vi "SDS Process Mngr.vi"(0 "State In":T5, 1 "Mngr Action":T12, 2 "FP":T11, 7 "Cartridges":T4, 9 "Manual Input":dbl format="%#_13g", 11 "error in (no error)":errorcluster, 12 "Config":T1={"Syringe size"=0, "Syringe address"=0, "# of ports"=0, "Init String"="Z0N1R", "Full Stroke (cnts)"=0, "Model"=enum."XC", "TW Position"=0.0, "Load Position"=0.0, "Bottom Position"=0.0, "Station ID"="", "Default Protocol"=path "", "Dry Time(s)"=0.0, "Python Version"="", "NFC SN Array"=["21121521200223", "21121521200186", "21121521200213", "52541737200062"], "Timing"={"Checking pres and leak"=0.0, "Priming input lines"=0.0, "Rinsing syringe"=0.0, "Filling well X w/ X"=0.0, "Drain well X"=0.0, "Clearing wells and lines"=0.0, "Draining wells"=0.0, "Rinsing all wells"=0.0, "Testing for leaks/clogs"=0.0, "Rinsing wells"=0.0}, "Pressure Specs"={"Pressure max"=0.0, "Pressure min"=0.0, "Decay delta"=0.0, "Pressure time"=0.0, "Conf. R"=0.0, "LeakRateMax"=0.0}}) -> (6 "State Out":T5, 15 "error out":errorcluster)   [LabVIEW 2020]
uses:
  Process Mngr.ctl
  Main Refs.ctl
  Wash Step.ctl
  Process State.ctl
  Results.ctl
  Vacuum Test.ctl
  Pressure Output.ctl
  Cartridge #.ctl
  Hardware/Tecan/Pump Config.ctl
  Timing Specs.ctl
  Vacuum Specs.ctl
  status update.ctl
  Cartridge Mngr.ctl
  Time elapsed.ctl
  Hardware/DAQ Mngr.ctl
  Lib/Time/Bottles.ctl
  Hardware/Mot Stage Mngr.ctl
  Update Single Cart.ctl
  Hardware/16CH Denkovi Mngr.ctl
  Hardware/Tricon Mngr.ctl
  Hardware/Tecan/Pump Control.ctl
  Pump Port.ctl
  Hardware/Tecan/Velocity Units.ctl
  Main Globals.vi
  Lib/Utilities.lvlib
panel:
  out "Reports":T6[](array[typedef])
  in  "Pressure Specs":T9
  out "Wash Array":T10[](array[typedef]) {"# of Rinses" max=10}
  # "Tecan Pump"
  # "Pressure"
  # "General"
  # "Timing"
  # "Protocol"
  # "Zaber"
  # "NFC Reader 1"
  # "NFC  Reader 2"
  # "NFC Reader 3"
  # "NFC Reader 4"
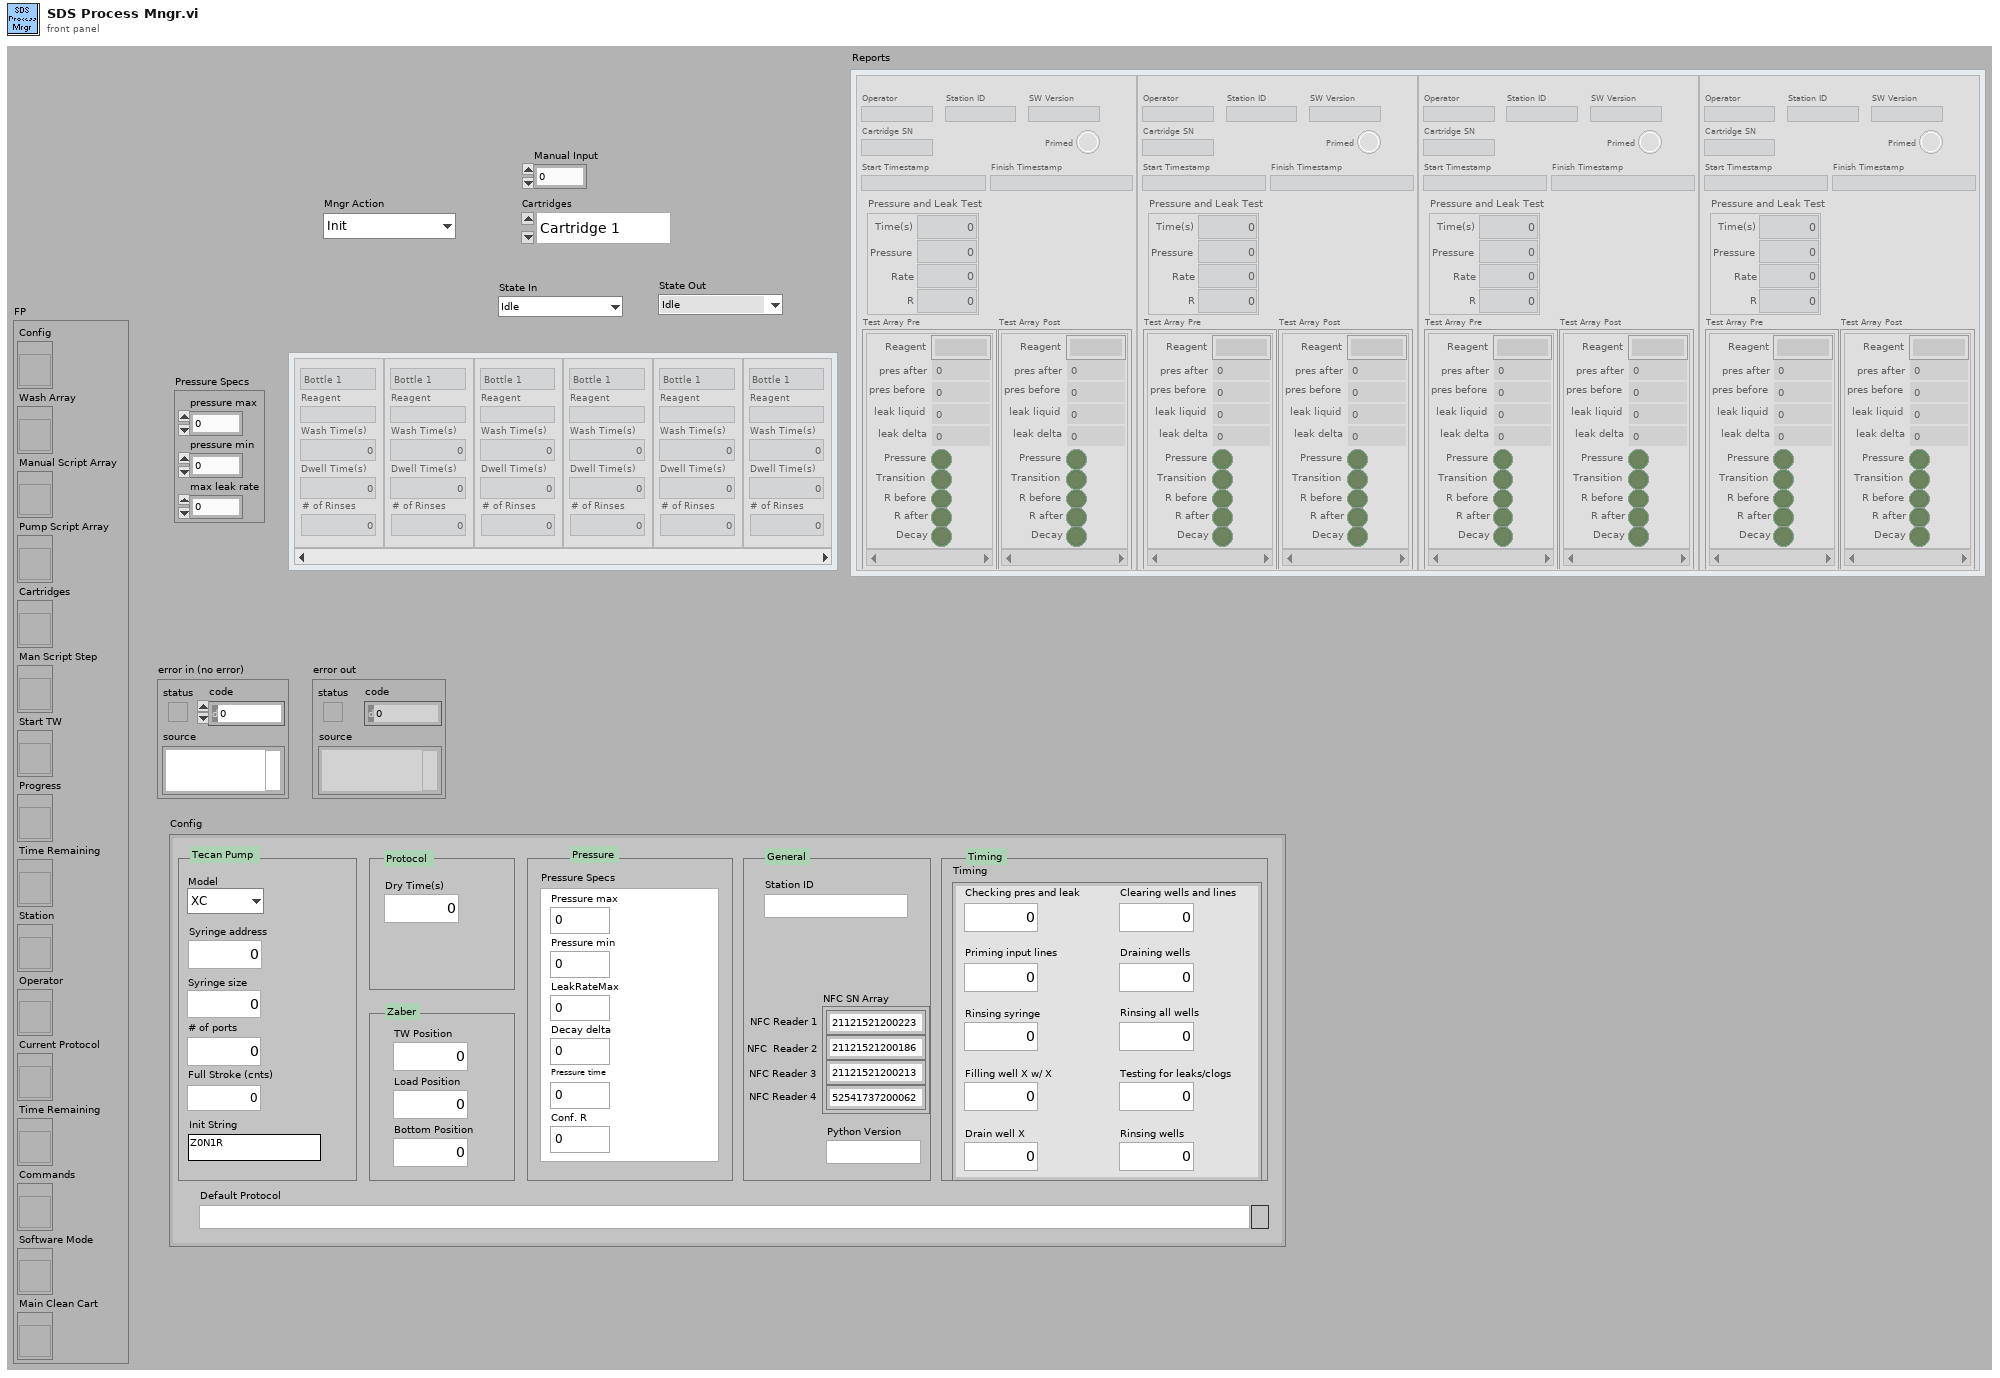
[diagram p1: front panel]
types:
  T1 = typedef "Pump Config.ctl" = cluster{"Syringe size":u32, "Syringe address":u32, "# of ports":u32, "Init String":string, "Full Stroke (cnts)":i32, "Model":enum16{"XC", "Centris"}, "TW Position":dbl, "Load Position":dbl, "Bottom Position":dbl, "Station ID":string, "Default Protocol":path, "Dry Time(s)":dbl, "Python Version":string, "NFC SN Array":string[], "Timing":T2, "Pressure Specs":T3}
  T2 = typedef "Timing Specs.ctl" = cluster{"Checking pres and leak":dbl, "Priming input lines":dbl, "Rinsing syringe":dbl, "Filling well X w/ X":dbl, "Drain well X":dbl, "Clearing wells and lines":dbl, "Draining wells":dbl, "Rinsing all wells":dbl, "Testing for leaks/clogs":dbl, "Rinsing wells":dbl}
  T3 = typedef "Vacuum Specs.ctl" = cluster{"Pressure max":dbl, "Pressure min":dbl, "Decay delta":dbl, "Pressure time":dbl, "Conf. R":dbl, "LeakRateMax":dbl}
  T4 = typedef "Cartridge #.ctl" = enum16{"Cartridge 1", "Cartridge 2", "Cartridge 3", "Cartridge 4"}
  T5 = typedef "Process State.ctl" = enum16{"Idle", "Init", "Check for SN", "Start TW", "SystemLeakTest", "Prime System", "Rinse Wells", "Fill Wells", "PrePresTest", "Apply Pressure", "PostPresTest", "Drain&Rinse", "Dry", "Report", "Finish", "Abort", "Error", "-rinse wells", "-check cartridge", "-clean cartridge", "-drain all", "-fill well"}
  T6 = typedef "Results.ctl" = cluster{"Operator":string, "Station ID":string, "SW Version":string, "Cartridge SN":string, "Primed":bool, "Start Timestamp":string, "Finish Timestamp":string, "Test Array Pre":T7[], "Test Array Post":T7[], "Pressure and Leak Test":T8}
  T7 = typedef "Vacuum Test.ctl" = cluster{"pres after":dbl, "pres before":dbl, "leak liquid":dbl, "leak delta":dbl, "Transition":bool, "Pressure":bool, "R before":bool, "R after":bool, "Reagent":string, "Decay":bool}
  T8 = typedef "Pressure Output.ctl" = cluster{"Time(s)":dbl, "Pressure":dbl, "Rate":dbl, "R":dbl}
  T9 = cluster{"pressure max":dbl, "pressure min":dbl, "max leak rate":dbl}
  T10 = typedef "Wash Step.ctl" = cluster{"Reagent":string, "Bottle":enum16{"Bottle 1", "Bottle 2", "Bottle 3", "Bottle 4"}, "Wash Time(s)":dbl, "Dwell Time(s)":dbl, "# of Rinses":i16}
  T11 = typedef "Main Refs.ctl" = cluster{"Config":refnum<vi>, "Wash Array":refnum<vi>, "Manual Script Array":refnum<vi>, "Pump Script Array":refnum<vi>, "Cartridges":refnum<vi>, "Man Script Step":refnum<vi>, "Start TW":refnum<vi>, "Progress":refnum<vi>, "Time Remaining":refnum<vi>, "Station":refnum<vi>, "Operator":refnum<vi>, "Current Protocol":refnum<vi>, "Time Remaining":refnum<vi>, "Commands":refnum<vi>, "Software Mode":refnum<vi>, "Main Clean Cart":refnum<vi>}
  T12 = typedef "Process Mngr.ctl" = enum16{"Init", "Run Step", "Update"}
  T13 = enum8{"Enabled", "Disabled", "Disabled and Grayed Out"}
  T14 = typedef "status update.ctl" = enum16{"Cartridge", "Main Status", "Reagent"}
  T15 = typedef "Cartridge Mngr.ctl" = enum16{"Init", "Update", "Detect", "Lock", "Read SN", "Unlock", "Error"}
  T16 = enum16{"Init Pressure", "Init Vacuum", "Save Pressure", "Save Vacuum", "Close"}
  T17 = typedef "DAQ Mngr.ctl" = enum16{"Init", "Read Pressure", "Read Vacuum", "Analyze Pres&Vac", "Analyze Vacuum", "Read Cartridges", "Lock Cartridge", "Unlock Cartridge", "Read PS", "Pinch Valve Engage", "Pinch Valve Disengage", "Close"}
  T18 = typedef "Time elapsed.ctl" = enum16{"Start", "Update", "Read"}
  T19 = typedef "Bottles.ctl" = enum16{"Bottle 1", "Bottle 2", "Bottle 3", "H2O", "Waste"}
  T20 = typedef "Mot Stage Mngr.ctl" = enum16{"Connect", "Init", "Status", "Send Cmd", "Current Pos", "Set Accel", "Set Max Vel", "Home", "Rel Move", "Abs Move", "Close"}
  T21 = typedef "Update Single Cart.ctl" = enum16{"Cart Status", "Cart Reagent"}
  T22 = typedef "16CH Denkovi Mngr.ctl" = enum16{"Search", "Init", "Set Peristaltic", "Set Pressure", "Set Vacuum", "Set PresVac", "Pres Vent&Close", "Vac Vent&Close", "Pres ON", "Vac ON", "Set All Relays", "Set One Relay", "Read Relays", "Close"}
  T23 = typedef "Pump Control.ctl" = cluster{"Syringe Pos":u32, "Rate":dbl, "Volume":dbl, "Valve":T24, "Action":enum32{"Withdraw", "Dispense", "Stop"}, "Move Type":enum32{"Abs", "Rel"}, "Init":bool, "Empty Syr.":bool, "Full Fill":bool, "Units":T25}
  T24 = typedef "Pump Port.ctl" = enum16{"Bottle 1", "Bottle 2", "Bottle 3", "Bottle 4", "Waste", "Well 1", "Well 2", "Well 3", "Well 4", "Bottle X", "Well X"}
  T25 = typedef "Velocity Units.ctl" = enum16{"ul/s", "ul/min"}
  T26 = typedef "Tricon Mngr.ctl" = enum16{"Init COM", "Set Config", "Init Pump", "Home", "Cmd", "Start Pump", "Set Valve", "Dispense", "Withdraw", "Status", "Close"}
  T27 = typedef "Cartridges.ctl" = cluster{"Cartridge 1":T28, "Cartridge 2":T28, "Cartridge 3":T28, "Cartridge 4":T28, "Current Status":string}
  T28 = typedef "Cartridge Status.ctl" = cluster{"Serial Number":string, "Reagent":string, "Cart Status":string, "Inserted":bool, "Eject":bool}
  T29 = typedef "Vacuum Output.ctl" = cluster{"Time(s)":dbl, "Vacuum":dbl, "Rate":dbl, "R":dbl}
  T30 = enum16{"Bottle 1", "Bottle 2", "Bottle 3", "Bottle 4"}
  T31 = typedef "Commands.ctl" = cluster{"Drain All Wells":bool, "Rinse All Wells":bool, "Prime":bool, "Well #":T32, "Bottle #":T19, "Fill":bool, "Run State":bool, "State":T5, "Empty Lines":bool, "Clean&Dry Cartridge":bool, "Check for leaks":bool, "Cart Test Array":T7[], "Number of rinses":dbl}
  T32 = typedef "Wells.ctl" = enum16{"Well 1", "Well 2", "Well 3", "Well 4"}
  T33 = cluster{"negative limit switch":bool, "positive limit switch":bool, "home switch":bool, "position marker":bool, "device enable":bool, "quick stop":bool, "general purpose J":bool, "general purpose I":bool, "general purpose H":bool, "general purpose G":bool, "general purpose F":bool, "general purpose E":bool, "general purpose D":bool, "general purpose C":bool, "general purpose B":bool, "general purpose A":bool}
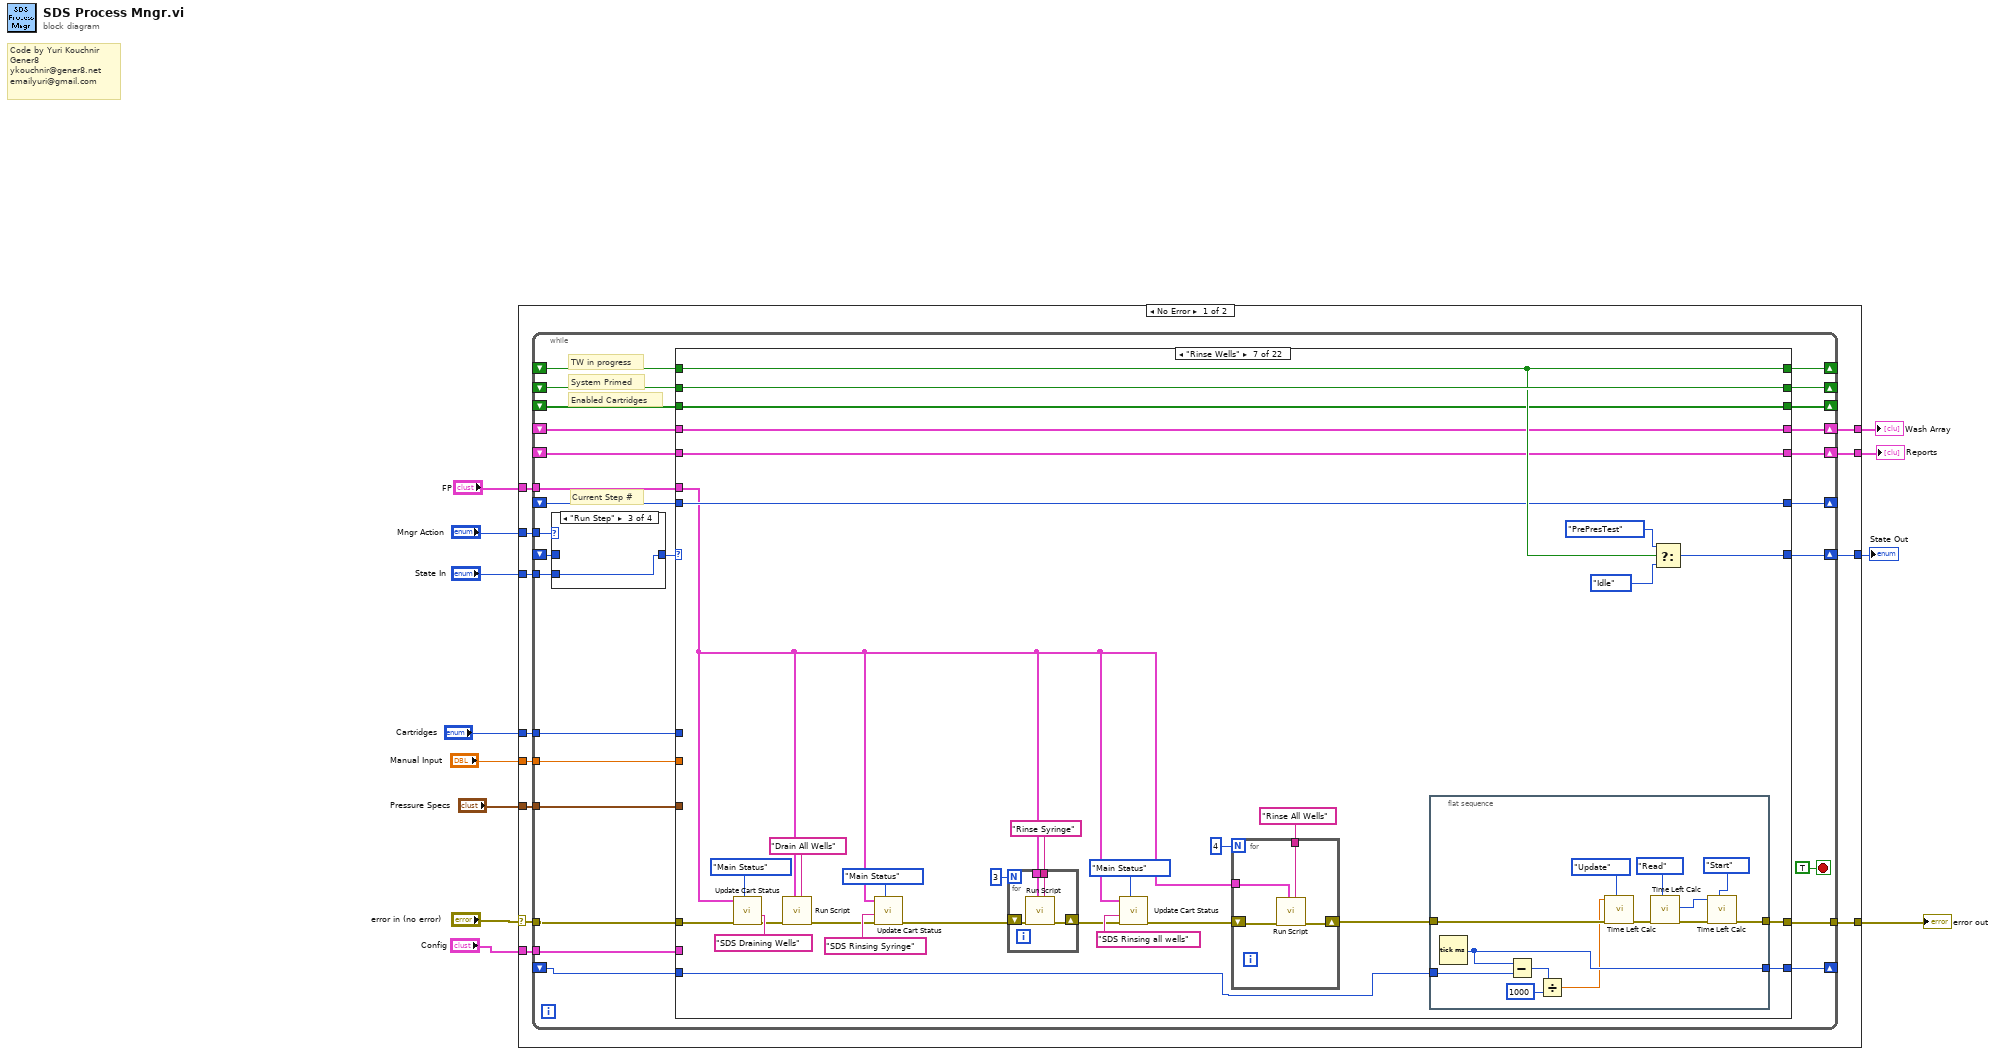
[diagram p0: block diagram]
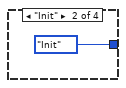
[diagram p3: hidden frame]
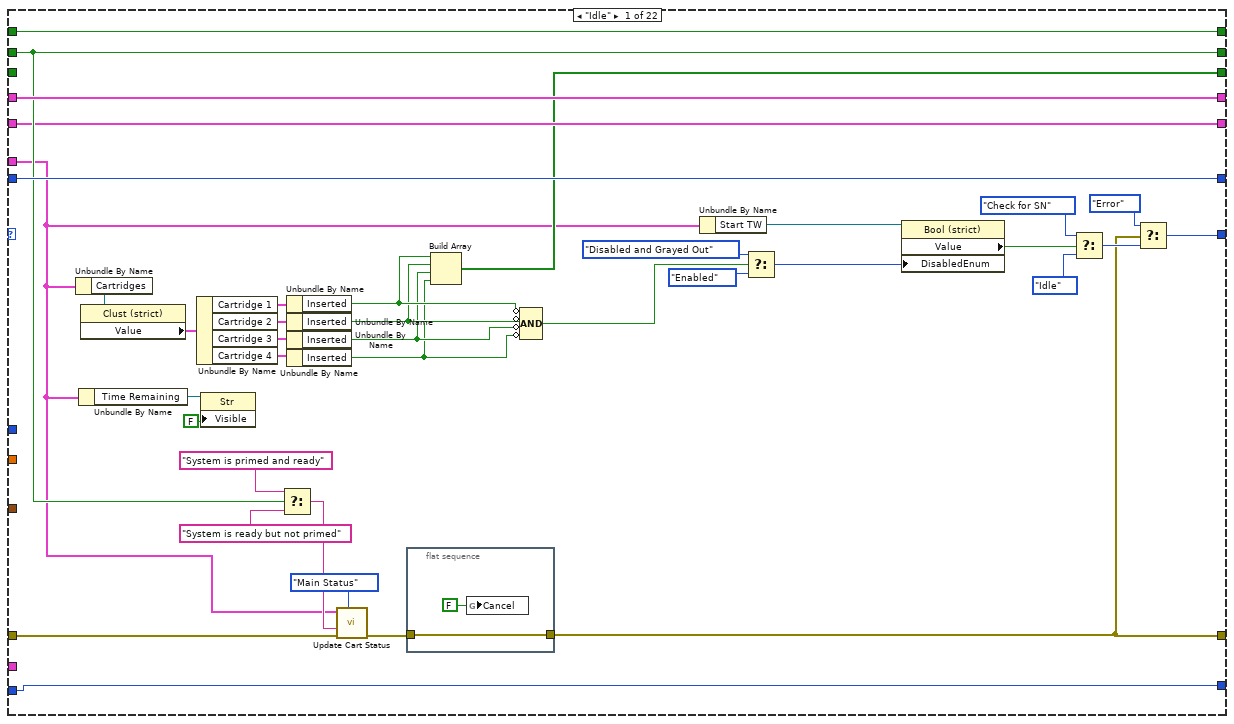
[diagram p5: hidden frame]
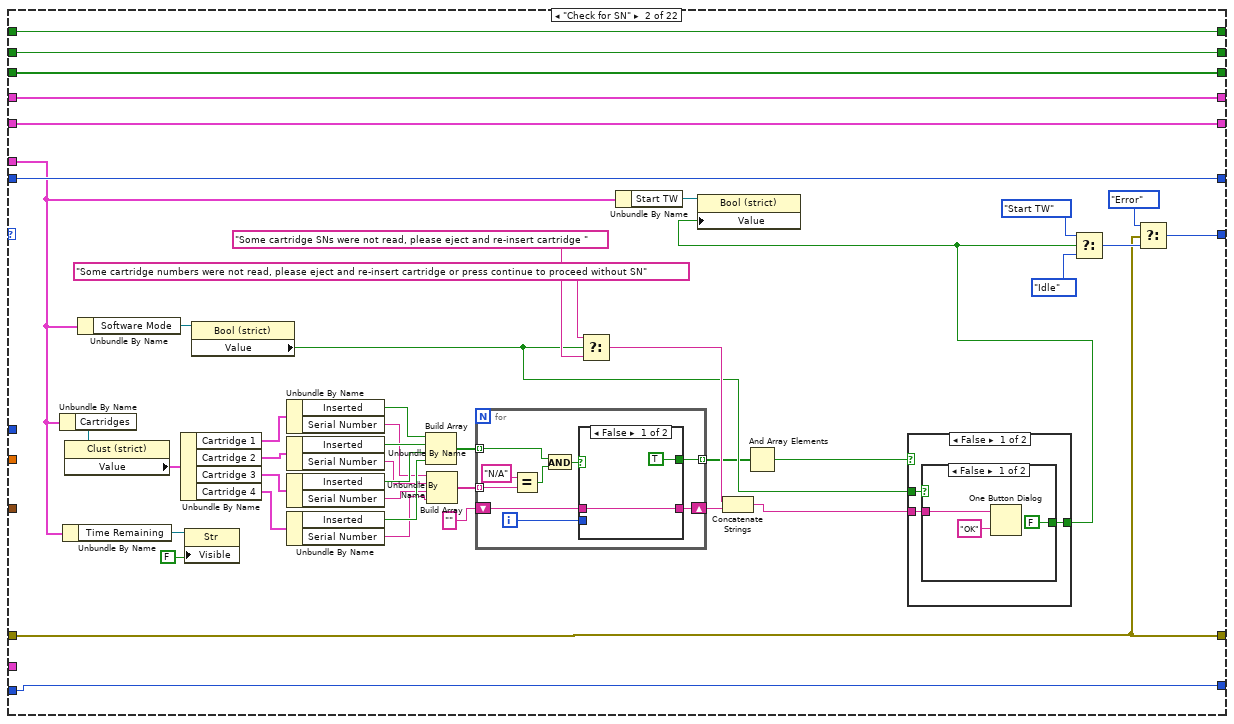
[diagram p6: hidden frame]
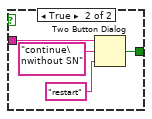
[diagram p7: hidden frame]
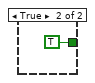
[diagram p8: hidden frame]
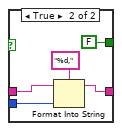
[diagram p9: hidden frame]
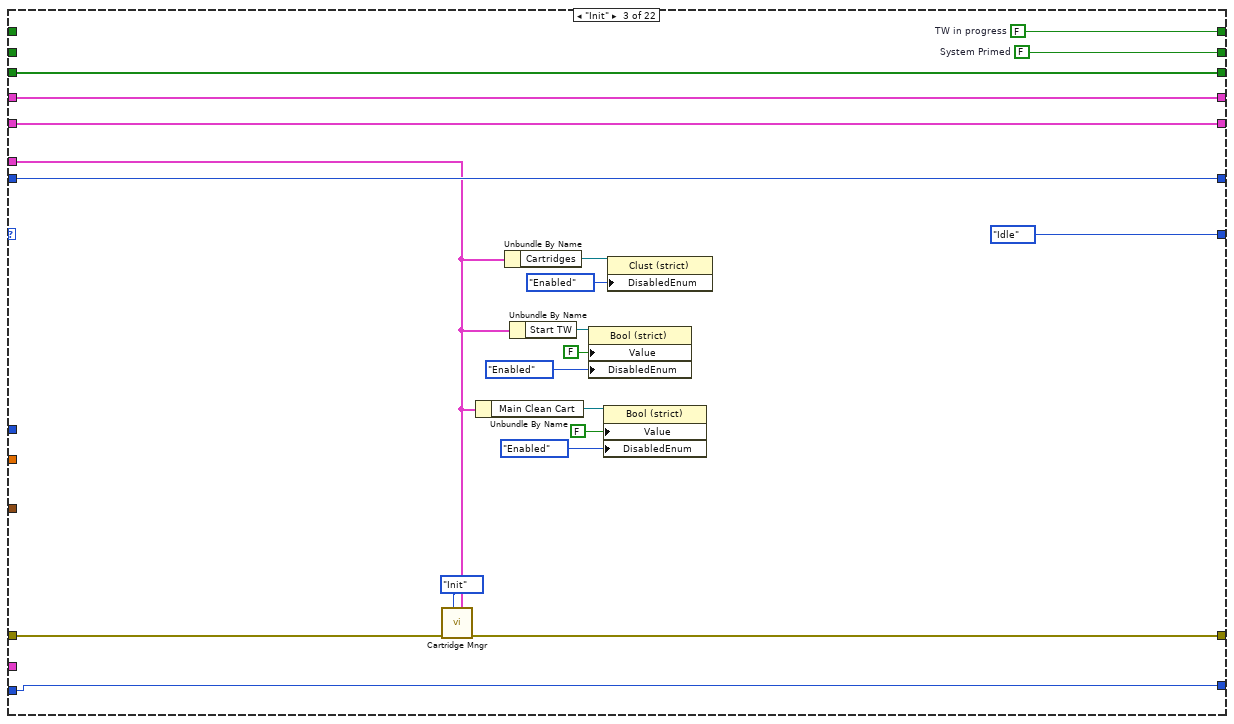
[diagram p10: hidden frame]
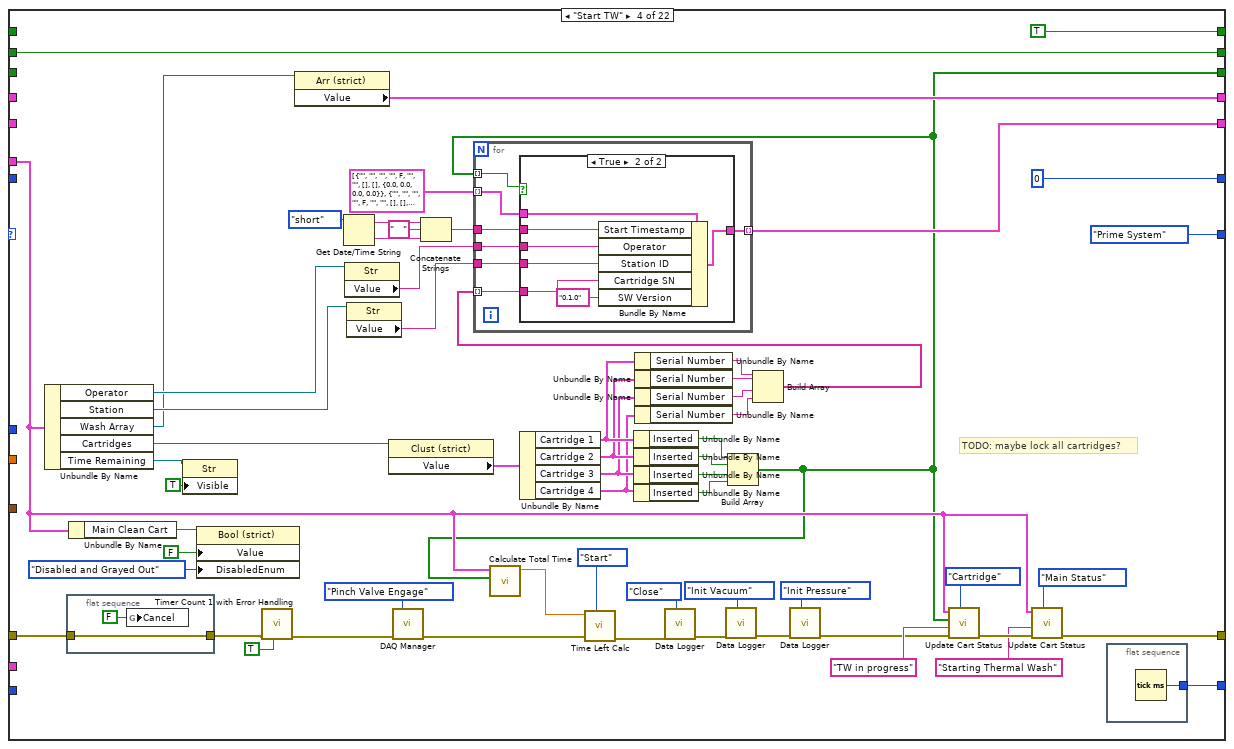
[diagram p11: hidden frame]
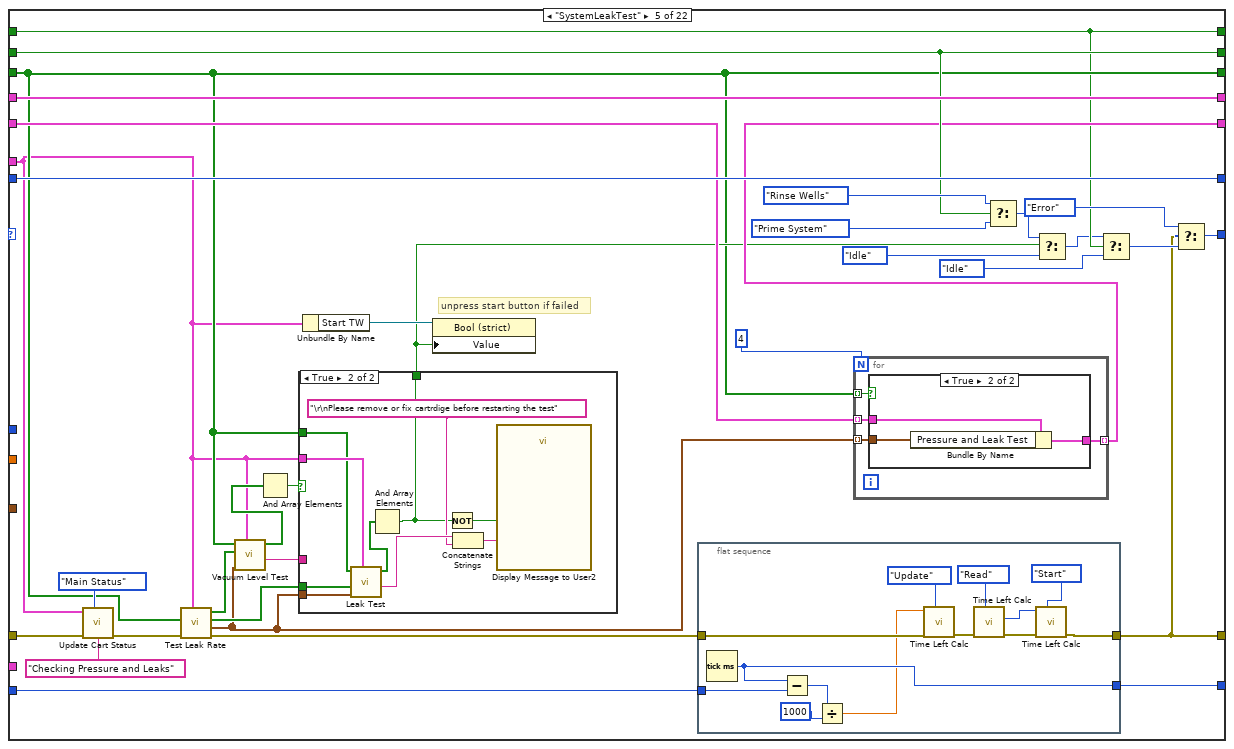
[diagram p13: hidden frame]
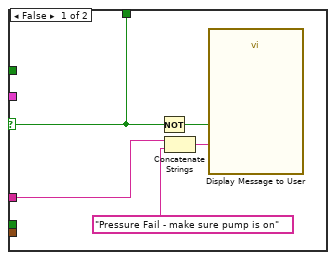
[diagram p14: hidden frame]
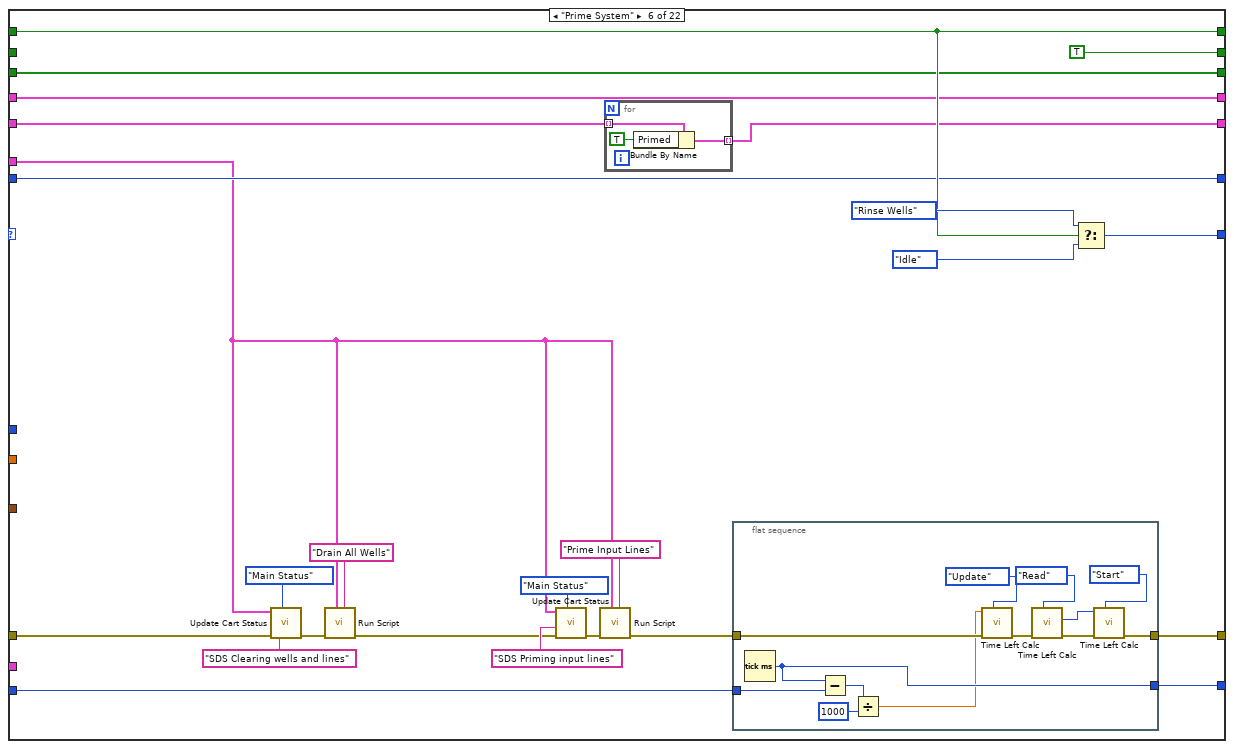
[diagram p16: hidden frame]
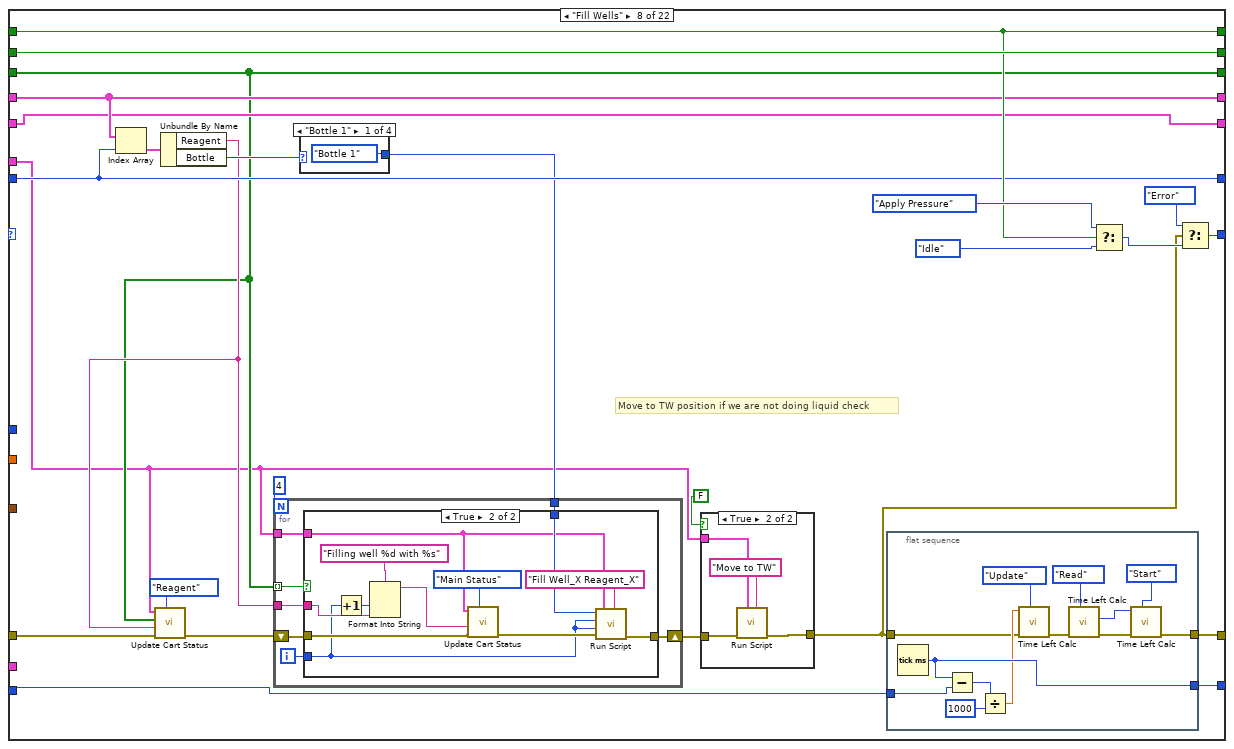
[diagram p17: hidden frame]
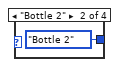
[diagram p19: hidden frame]
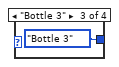
[diagram p20: hidden frame]
diagram:
  # "Code by Yuri Kouchnir\nGener8\nykouchnir@gener8.net\nemailyuri@gmail.com"
  n1 = case shown="No Error" "error in (no error)" {
    selector: "error in (no error)" -> [w24 w1289]
    tunnel: [w23 w1289] -> w11
    tunnel: "Mngr Action" -> [w22 _]
    tunnel: "FP" -> [w21 _]
    tunnel: "Pressure Specs" -> [w20 _]
    tunnel: [w19 _] -> w7
    tunnel: [w18 _] -> w6
    tunnel: [w17 _] -> w4
    tunnel: "State In" -> [w16 _]
    tunnel: "Cartridges" -> [w15 _]
    tunnel: "Manual Input" -> [w14 _]
    tunnel: "Config" -> [w13 _]
    frame No Error {
      n2 = while {
        tunnel: w24 -> [w50]
        tunnel: [w49] -> w23
        tunnel: w22 -> [w44]
        shift-right: [w48] -> w19
        shift-left: _ -> [w46]
        tunnel: w21 -> [w47]
        shift-right: [w43] -> _
        shift-left: _ -> [w42]
        shift-right: [w41] -> w18
        shift-left: _ -> [w40]
        shift-right: [w39] -> _
        shift-left: _ -> [w38]
        shift-right: [w37] -> _
        shift-left: _ -> [w36]
        shift-right: [w35] -> _
        shift-left: _ -> [w34]
        tunnel: w20 -> [w33]
        shift-right: [w32] -> w17
        shift-left: _ -> [w31]
        tunnel: w16 -> [w30]
        tunnel: w15 -> [w29]
        tunnel: w14 -> [w28]
        shift-right: [w27] -> _
        shift-left: _ -> [w26]
        tunnel: w13 -> [w25]
        stop <- TRUE stop-if-true
        # "Current Step #"
        # "Enabled Cartridges"
        # "System Primed"
        # "TW in progress"
        n3 = case shown="\"Run Step\"" w44 {
          tunnel: w46 -> [w52 _ _ w55]
          tunnel: [w52 Process_State."Init" ("State") w54 w55] -> w45
          tunnel: w30 -> [_ _ w54 _]
          frame Default {
          }
          frame "Init" {
          }
          frame "Run Step" {
          }
          frame "Update" {
          }
        }
        n4 = case shown="\"Rinse Wells\"" w45 {
          tunnel: w50 -> [w63 w104 w167 w215 w296 w339 w396 w436 w522 w609 w679 w759 w876 w926 w962 w979 w1041 w1059 w1092 w1115 w1176 w1249]
          tunnel: [w61 w104 w180 w236 w269 w342 w378 w431 w506 w599 w668 w751 w864 w925 w954 w981 w1033 w1050 w1084 w1109 w1163 w1231] -> w49
          tunnel: [w84 w131 Process_State."Idle" ("State") Process_State."Prime System" ("State") w293 w359 w406 w446 w525 w624 w682 w781 w884 Process_State."Idle" ("State") Process_State."Idle" ("State") Process_State."Finish" ("State") Process_State."Idle" ("State") w1069 w1100 w1123 w1179 w1252] -> w48
          tunnel: w47 -> [w58 w106 w169 w197 w270 w344 w380 w432 w513 w597 w671 w760 w868 w928 w945 w977 w1024 w1052 w1095 w1118 w1146 w1236]
          tunnel: [w82 w130 w185 w213 w291 TRUE ("System Primed") w403 w451 w527 w628 w685 w786 w896 w941 w972 w992 w1047 w1071 w1104 w1127 w1166 w1238] -> w43
          tunnel: w42 -> [w82 w130 _ w213 w291 _ w403 w451 w527 w628 w685 w786 w896 w941 w972 w992 w1047 w1071 w1104 w1127 w1166 w1238]
          tunnel: [w91 w137 w181 w204 w298 w353 w399 w441 w524 w615 w681 w777 w883 w940 w971 w991 w1046 w1068 w1098 w1121 w1178 w1251] -> w41
          tunnel: w40 -> [w91 w137 w181 _ w298 w353 w399 w441 w524 w615 w681 w777 w883 w940 w971 w991 w1046 w1068 w1098 w1121 w1178 w1251]
          tunnel: [w93 w139 w184 TRUE ("TW in progress") w274 w356 w402 w449 w511 w627 w666 w755 w879 w939 FALSE ("TW in progress") w990 FALSE ("TW in progress") w1056 w1103 w1126 w1172 w1245] -> w39
          tunnel: w38 -> [w93 w139 _ _ w274 w356 w402 w449 w511 w627 w666 w755 w879 w939 _ w990 _ w1056 w1103 w1126 w1172 w1245]
          tunnel: [w92 w138 w182 0 w297 w354 w400 w445 w518 w621 w675 w778 w880 w938 w970 w989 w1045 w1055 w1099 w1122 w1173 w1246] -> w37
          tunnel: w36 -> [w92 w138 w182 _ w297 w354 w400 w445 w518 w621 w675 w779 w880 w938 w970 w989 w1045 w1055 w1099 w1122 w1173 w1246]
          tunnel: [w64 w116 w183 w196 w275 w355 w401 w434 w499 w605 w670 w765 w867 w937 w969 w975 w1042 w1049 w1096 w1119 w1130 w1226] -> w35
          tunnel: w34 -> [_ w116 w183 _ w275 w355 w401 w434 w510 w605 w657 w765 w867 w937 w969 w975 w1042 w1049 w1096 w1119 w1130 w1226]
          tunnel: w33 -> [_ _ _ _ _ _ _ _ _ w617 _ _ w891 _ _ _ _ _ _ _ _ _]
          tunnel: [w78 w129 w173 w229 w283 w349 w382 w439 w516 w612 w673 w775 w878 w927 w968 w980 w1031 w1067 w1097 w1120 w1147 w1230] -> w32
          tunnel: w31 -> [w78 w129 w173 _ w285 w350 w382 w439 w517 w612 w674 w775 w878 w927 w968 w982 w1031 w1067 w1097 w1120 w1147 w1230]
          tunnel: w29 -> [_ _ _ _ _ _ _ _ _ _ _ _ _ _ _ _ _ _ _ _ _ _]
          tunnel: w28 -> [_ _ _ _ _ _ _ _ _ _ _ _ _ _ _ _ _ w1054 _ _ _ _]
          tunnel: [w56 w96 w168 w195 w266 w340 w376 w430 w503 w598 w659 w750 w862 w924 w953 w974 w1023 w1048 w1083 w1107 w1145 w1224] -> w27
          tunnel: w26 -> [w56 w96 w168 _ w268 w343 w379 w428 w502 _ w658 w749 _ w924 w953 w974 w1023 w1048 w1083 w1107 w1145 w1224]
          tunnel: w25 -> [_ _ _ _ _ _ _ _ _ _ _ _ _ _ w951 _ _ _ _ _ _ _]
          frame "Idle" {
            n5 = Unbundle By Name(w58) -> ("Cartridges"=w73:refnum<vi>)
            n6 = Unbundle By Name(w58) -> ("Time Remaining"=w60:refnum<vi>)
            n7 = property class="Clust (strict)"(reference=w73) -> ("Value"=w77:T27)  [unwired: 1 in, 2 out]
            n8 = Unbundle By Name(w77) -> ("Cartridge 1"=w72:T28, "Cartridge 2"=w76:T28, "Cartridge 3"=w75:T28, "Cartridge 4"=w74:T28)
            n9 = property class="Str"(reference=w60, "Visible"=FALSE) -> ()  [unwired: 1 in, 2 out]
            n10 = Select(t="System is primed and ready" ("Reagent"), s=w82, f="System is ready but not primed" ("Reagent")) -> (s? t:f=w79:string)
            n11 = Unbundle By Name(w72) -> ("Inserted"=w68:bool)
            n12 = Unbundle By Name(w76) -> ("Inserted"=w67:bool)
            n13 = Unbundle By Name(w75) -> ("Inserted"=w66:bool)
            n14 = Unbundle By Name(w74) -> ("Inserted"=w65:bool)
            n15 = call "Update Cart Status.vi"("Selection"=status_update."Main Status", "error in (no error)"=w63, "String"=w79, "FP"=w58) -> ("error out"=w62:errorcluster)  [unwired: 7 in]
            n16 = flat-sequence {
              tunnel: w62 -> [w95]
              tunnel: [w95] -> w61
              frame #0 {
                n17 = global write "Main Globals.vi" "Cancel"(FALSE ("Cancel")) -> ()
              }
            }
            n18 = Build Array(w68, w67, w66, w65) -> (w64:bool[])
            n19 = Compound Arithmetic op=AND(invert w68, invert w67, invert w66, invert w65) -> (w57:bool)
            n20 = Unbundle By Name(w58) -> ("Start TW"=w90:refnum<vi>)
            n21 = Select(t=T13."Disabled and Grayed Out" ("Disabled"), s=w57, f=T13."Enabled" ("Disabled")) -> (s? t:f=w69:T13)
            n22 = property class="Bool (strict)"(reference=w90, "DisabledEnum"=w69) -> ("Value"=w89:bool)  [unwired: 1 in, 2 out]
            n23 = Select(t=Process_State."Check for SN" ("State"), s=w89, f=Process_State."Idle" ("State")) -> (s? t:f=w86:T5)
            n24 = Select(t=Process_State."Error" ("State"), s=w61, f=w86) -> (s? t:f=w84:T5)
          }
          frame "Check for SN" {
            n25 = Unbundle By Name(w106) -> ("Cartridges"=w124:refnum<vi>)
            n26 = Unbundle By Name(w106) -> ("Time Remaining"=w118:refnum<vi>)
            n27 = property class="Clust (strict)"(reference=w124) -> ("Value"=w128:T27)  [unwired: 1 in, 2 out]
            n28 = Unbundle By Name(w106) -> ("Software Mode"=w105:refnum<vi>)
            n29 = Unbundle By Name(w128) -> ("Cartridge 1"=w123:T28, "Cartridge 2"=w127:T28, "Cartridge 3"=w126:T28, "Cartridge 4"=w125:T28)
            n30 = property class="Str"(reference=w118, "Visible"=FALSE) -> ()  [unwired: 1 in, 2 out]
            n31 = property class="Bool (strict)"(reference=w105) -> ("Value"=w100:bool)  [unwired: 1 in, 2 out]
            n32 = Unbundle By Name(w123) -> ("Inserted"=w122:bool, "Serial Number"=w115:string)
            n33 = Unbundle By Name(w127) -> ("Inserted"=w121:bool, "Serial Number"=w114:string)
            n34 = Unbundle By Name(w126) -> ("Inserted"=w120:bool, "Serial Number"=w113:string)
            n35 = Unbundle By Name(w125) -> ("Inserted"=w119:bool, "Serial Number"=w112:string)
            n36 = Build Array(w122, w121, w120, w119) -> (w111:bool[])
            n37 = Build Array(w115, w114, w113, w112) -> (w110:string[])
            n38 = for {
              tunnel: w111 -> [w154] mode=indexing
              tunnel: w110 -> [w157] mode=indexing
              shift-right: [w152] -> w107
              shift-left: "" ("Serial Number") -> [w158]
              tunnel: [w151] -> w99 mode=indexing
              i -> [w159]
              n39 = Equal?(x="N/A", y=w157) -> (x = y?=w155:bool)
              n40 = And(x=w154, y=w155) -> (x .and. y?=w153:bool)
              n41 = case shown="False" w153 {
                tunnel: w159 -> [_ w166]
                tunnel: w158 -> [w161 w165]
                tunnel: [w161 w164] -> w152
                tunnel: [TRUE FALSE] -> w151
                frame False {
                }
                frame True {
                  n42 = Format Into String(format string="%d,", initial string=w165, w166) -> (resulting string=w164:string)  [unwired: 1 in, 1 out]
                }
              }
            }
            n43 = Select(t="Some cartridge numbers were not read, please eject and re-insert cartridge or press continue to proceed without SN" ("message"), s=w100, f="Some cartridge SNs were not read, please eject and re-insert cartridge " ("message")) -> (s? t:f=w101:string)
            n44 = Unbundle By Name(w106) -> ("Start TW"=w136:refnum<vi>)
            n45 = Concatenate Strings(w101, w107) -> (w108:string)
            n46 = And Array Elements(Boolean array=w99) -> (logical AND=w98:bool)
            n47 = case shown="False" w98 {
              tunnel: w108 -> [w142 _]
              tunnel: w100 -> [w141 _]
              tunnel: [w140 TRUE ("T button?")] -> w97
              frame False {
                n48 = case shown="False" w141 {
                  tunnel: w142 -> [w144 w149]
                  tunnel: [FALSE ("T button?") w146] -> w140
                  frame False {
                    n49 = One Button Dialog(message=w144, button name ("OK")="OK") -> ()  [unwired: 1 out]
                  }
                  frame True {
                    n50 = Two Button Dialog(message=w149, 1:"restart" ("T button name (\"OK\")"), 2:"continue\nwithout SN" ("T button name (\"OK\")")) -> (T button?=w146:bool)
                  }
                }
              }
              frame True {
              }
            }
            n51 = property class="Bool (strict)"(reference=w136, "Value"=w97) -> ()  [unwired: 1 in, 2 out]
            n52 = Select(t=Process_State."Start TW" ("State"), s=w97, f=Process_State."Idle" ("State")) -> (s? t:f=w133:T5)
            n53 = Select(t=Process_State."Error" ("State"), s=w104, f=w133) -> (s? t:f=w131:T5)
          }
          frame "Init" {
            w184 = FALSE  # TW in progress
            w185 = FALSE  # System Primed
            n54 = call "Cartridge Mngr.vi"("Main References"=w169, "Mngr Action"=Cartridge_Mngr."Init", "error in (no error)"=w167) -> ("error out"=w180:errorcluster)  [unwired: 6 in, 2 out]
            n55 = Unbundle By Name(w169) -> ("Main Clean Cart"=w170:refnum<vi>)
            n56 = Unbundle By Name(w169) -> ("Cartridges"=w178:refnum<vi>)
            n57 = Unbundle By Name(w169) -> ("Start TW"=w176:refnum<vi>)
            n58 = property class="Bool (strict)"(reference=w176, "Value"=FALSE, "DisabledEnum"=T13."Enabled" ("Disabled")) -> ()  [unwired: 1 in, 2 out]
            n59 = property class="Bool (strict)"(reference=w170, "Value"=FALSE, "DisabledEnum"=T13."Enabled" ("Disabled")) -> ()  [unwired: 1 in, 2 out]
            n60 = property class="Clust (strict)"(reference=w178, "DisabledEnum"=T13."Enabled" ("Disabled")) -> ()  [unwired: 1 in, 2 out]
          }
          frame "Start TW" {
            # "TODO: maybe lock all cartridges?"
            n61 = Unbundle By Name(w197) -> ("Operator"=w219:refnum<vi>, "Station"=w217:refnum<vi>, "Wash Array"=w208:refnum<vi>, "Cartridges"=w214:refnum<vi>, "Time Remaining"=w202:refnum<vi>)
            n62 = flat-sequence {
              tunnel: w215 -> [w250]
              tunnel: [w250] -> w210
              frame #0 {
                n63 = global write "Main Globals.vi" "Cancel"(FALSE ("Cancel")) -> ()
              }
            }
            n64 = Unbundle By Name(w197) -> ("Main Clean Cart"=w198:refnum<vi>)
            n65 = property class="Str"(reference=w202, "Visible"=TRUE) -> ()  [unwired: 1 in, 2 out]
            n66 = property class="Bool (strict)"(reference=w198, "Value"=FALSE, "DisabledEnum"=T13."Disabled and Grayed Out" ("Disabled")) -> ()  [unwired: 1 in, 2 out]
            n67 = call "Timer Count 1 with Error Handling.vi"("Reset"=TRUE, "error in (no error)"=w210) -> ("error out"=w193:errorcluster)  [unwired: 6 in, 3 out]
            n68 = property class="Arr (strict)"(reference=w208) -> ("Value"=w204:T10[])  [unwired: 1 in, 2 out]
            n69 = Get Date/Time String(date format (0)=enum16{"short", "long", "abbreviated"}."short") -> (date string=w233:string, time string=w232:string)  [unwired: 2 in]
            n70 = property class="Str"(reference=w219) -> ("Value"=w218:string)  [unwired: 1 in, 2 out]
            n71 = property class="Str"(reference=w217) -> ("Value"=w216:string)  [unwired: 1 in, 2 out]
            n72 = property class="Clust (strict)"(reference=w214) -> ("Value"=w212:T27)  [unwired: 1 in, 2 out]
            n73 = call "DAQ Manager.vi"("DAQ Mngr Action"=DAQ_Mngr."Pinch Valve Engage", "error in (no error)"=w193) -> ("error out"=w192:errorcluster)  [unwired: 6 in, 7 out]
            n74 = Concatenate Strings(w233, "   " ("string"), w232) -> (w230:string)
            n75 = Unbundle By Name(w212) -> ("Cartridge 1"=w228:T28, "Cartridge 2"=w227:T28, "Cartridge 3"=w226:T28, "Cartridge 4"=w225:T28)
            n76 = Unbundle By Name(w228) -> ("Inserted"=w245:bool)
            n77 = Unbundle By Name(w227) -> ("Inserted"=w244:bool)
            n78 = Unbundle By Name(w226) -> ("Inserted"=w243:bool)
            n79 = Unbundle By Name(w225) -> ("Inserted"=w242:bool)
            n80 = Unbundle By Name(w228) -> ("Serial Number"=w224:string)
            n81 = Unbundle By Name(w227) -> ("Serial Number"=w223:string)
            n82 = Unbundle By Name(w226) -> ("Serial Number"=w222:string)
            n83 = Unbundle By Name(w225) -> ("Serial Number"=w221:string)
            n84 = Build Array(w245, w244, w243, w242) -> (w196:bool[])
            n85 = call "Calculate Total Time.vi"("Boolean array"=w196, "FP"=w197) -> ("Total Time(s)"=w203:dbl)  [unwired: 9 in]
            n86 = call "Time Left Calc.vi"("Enum"=Time_elapsed."Start", "error in (no error)"=w192, "Time"=w203) -> ("error out"=w206:errorcluster)  [unwired: 6 in, 2 out]
            n87 = call "Data Logger.vi"("Action"=T16."Close", "error in"=w206) -> ("error out"=w207:errorcluster)  [unwired: 9 in]
            n88 = call "Data Logger.vi"("Action"=T16."Init Vacuum", "error in"=w207) -> ("error out"=w191:errorcluster)  [unwired: 9 in]
            n89 = Build Array(w224, w223, w222, w221) -> (w220:string[])
            n90 = for {
              tunnel: T6[] [{"Operator"="", "Station ID"="", "SW Version"="", "Cartridge SN"="", "Primed"=FALSE, "Start Timestamp"="", "Finish Timestamp"="", "Test Array Pre"=[], "Test Array Post"=[], "Pressure and Leak Test"={"Time(s)"=0.0, "Pressure"=0.0, "Rate"=0.0, "R"=0.0}}, {"Operator"="", "Station ID"="", "SW Version"="", "Cartridge SN"="", "Primed"=FALSE, "Start Timestamp"="", "Finish Timestamp"="", "Test Array Pre"=[], "Test Array Post"=[], "Pressure and Leak Test"={"Time(s)"=0.0, "Pressure"=0.0, "Rate"=0.0, "R"=0.0}}, {"Operator"="", "Station ID"="", "SW Version"="", "Cartridge SN"="", "Primed"=FALSE, "Start Timestamp"="", "Finish Timestamp"="", "Test Array Pre"=[], "Test Array Post"=[], "Pressure and Leak Test"={"Time(s)"=0.0, "Pressure"=0.0, "Rate"=0.0, "R"=0.0}}, {"Operator"="", "Station ID"="", "SW Version"="", "Cartridge SN"="", "Primed"=FALSE, "Start Timestamp"="", "Finish Timestamp"="", "Test Array Pre"=[], "Test Array Post"=[], "Pressure and Leak Test"={"Time(s)"=0.0, "Pressure"=0.0, "Rate"=0.0, "R"=0.0}}] ("Reports") -> [w257] mode=indexing
              tunnel: w230 -> [w256]
              tunnel: [w255] -> w229 mode=indexing
              tunnel: w196 -> [w254] mode=indexing
              tunnel: w220 -> [w253] mode=indexing
              tunnel: w218 -> [w252]
              tunnel: w216 -> [w251]
              n91 = case shown="True" w254 {
                tunnel: w257 -> [w258 w265]
                tunnel: w256 -> [_ w264]
                tunnel: [w258 w263] -> w255
                tunnel: w253 -> [_ w262]
                tunnel: w252 -> [_ w261]
                tunnel: w251 -> [_ w260]
                frame False {
                }
                frame True {
                  n92 = Bundle By Name(cluster=w265, "Start Timestamp"=w264, "Operator"=w261, "Station ID"=w260, "Cartridge SN"=w262, "SW Version"="0.1.0") -> (w263:T6)
                }
              }
            }
            n93 = call "Data Logger.vi"("Action"=T16."Init Pressure", "error in"=w191) -> ("error out"=w190:errorcluster)  [unwired: 9 in]
            n94 = call "Update Cart Status.vi"("Selection"=status_update."Cartridge", "error in (no error)"=w190, "String"="TW in progress" ("Reagent"), "Array"=w196, "FP"=w197) -> ("error out"=w240:errorcluster)  [unwired: 6 in]
            n95 = call "Update Cart Status.vi"("Selection"=status_update."Main Status", "error in (no error)"=w240, "String"="Starting Thermal Wash" ("Reagent"), "FP"=w197) -> ("error out"=w236:errorcluster)  [unwired: 7 in]
            n96 = flat-sequence {
              tunnel: [w248] -> w195
              frame #0 {
                n97 = Tick Count (ms)() -> (millisecond timer value=w248:u32)
              }
            }
          }
          frame "SystemLeakTest" {
            # "unpress start button if failed"
            n98 = call "Update Cart Status.vi"("Selection"=status_update."Main Status", "String"="Checking Pressure and Leaks" ("Reagent"), "FP"=w270) -> ()  [unwired: 8 in, 1 out]
            n99 = call "Test Leak Rate.vi"("Main References"=w270, "error in (no error)"=w296, "Cart Array"=w275) -> ("error out"=w267:errorcluster, "Results"=w277:T29[], "RatePass"=w278:bool[], "Pres Pass"=w282:bool[])  [unwired: 5 in]
            n100 = call "Vacuum Level Test.vi"("FP"=w270, "Results"=w277, "Pres Pass"=w282, "Cart Array"=w275) -> ("Error String"=w280:string, "Pass/Fail Array"=w276:bool[])  [unwired: 6 in]
            n101 = And Array Elements(Boolean array=w276) -> (logical AND=w281:bool)
            n102 = case shown="True" w281 {
              selector: w281 -> [w312 _]
              tunnel: w280 -> [w314 _]
              tunnel: [w312 w319] -> w279
              tunnel: w278 -> [_ w326]
              tunnel: w270 -> [_ w325]
              tunnel: w277 -> [_ w324]
              tunnel: w275 -> [_ w318]
              frame False {
                n103 = Not(x=w312) -> (.not. x?=w316:bool)
                n104 = Concatenate Strings(w314, "Pressure Fail - make sure pump is on" ("string")) -> (w315:string)
                n105 = call "Display Message to User"("Enable"=w316, "Message"=w315) -> ()  [unwired: 8 in, 2 out]
              }
              frame True {
                n106 = call "Leak Test.vi"("FP"=w325, "Results"=w324, "RatePass"=w326, "Cart Array"=w318) -> ("Error String"=w323:string, "Pass/Fail Array"=w317:bool[])  [unwired: 6 in]
                n107 = And Array Elements(Boolean array=w317) -> (logical AND=w319:bool)
                n108 = Not(x=w319) -> (.not. x?=w322:bool)
                n109 = Concatenate Strings(w323, "\r\nPlease remove or fix cartrdige before restarting the test" ("string")) -> (w321:string)
                n110 = call "Display Message to User2"("Enable"=w322, "Message"=w321) -> ()  [unwired: 8 in, 2 out]
              }
            }
            n111 = Unbundle By Name(w270) -> ("Start TW"=w288:refnum<vi>)
            n112 = property class="Bool (strict)"(reference=w288, "Value"=w279) -> ()  [unwired: 1 in, 2 out]
            n113 = flat-sequence {
              tunnel: [w308] -> w269
              tunnel: w268 -> [w307]
              tunnel: w267 -> [w305]
              tunnel: [w302] -> w266
              frame #0 {
                n114 = Tick Count (ms)() -> (millisecond timer value=w302:u32)
                n115 = Subtract(x=w302, y=w307) -> (x-y=w299:u32)
                n116 = Divide(x=w299, y=u32 1000) -> (x/y=w301:dbl)
                n117 = call "Time Left Calc.vi"("Enum"=Time_elapsed."Update", "error in (no error)"=w305, "Time"=w301) -> ("error out"=w304:errorcluster)  [unwired: 6 in, 2 out]
                n118 = call "Time Left Calc.vi"("Enum"=Time_elapsed."Read", "error in (no error)"=w304) -> ("error out"=w310:errorcluster, "Time Left"=w309:u32)  [unwired: 7 in, 1 out]
                n119 = call "Time Left Calc.vi"("Enum"=Time_elapsed."Start", "error in (no error)"=w310, "Time"=w309) -> ("error out"=w308:errorcluster)  [unwired: 6 in, 2 out]
              }
            }
            n120 = for {
              N: 4 -> [_]
              tunnel: w285 -> [w329] mode=indexing
              tunnel: w275 -> [w330] mode=indexing
              tunnel: w277 -> [w328] mode=indexing
              tunnel: [w327] -> w283 mode=indexing
              n121 = case shown="True" w330 {
                tunnel: w329 -> [w331 w334]
                tunnel: w328 -> [_ w333]
                tunnel: [w331 w332] -> w327
                frame False {
                }
                frame True {
                  n122 = Bundle By Name(cluster=w334, "Pressure and Leak Test"=w333) -> (w332:T6)
                }
              }
            }
            n123 = Select(t=Process_State."Rinse Wells" ("State"), s=w291, f=Process_State."Prime System" ("State")) -> (s? t:f=w290:T5)
            n124 = Select(t=w290, s=w279, f=Process_State."Idle") -> (s? t:f=w273:T5)
            n125 = Select(t=w273, s=w274, f=Process_State."Idle") -> (s? t:f=w271:T5)
            n126 = Select(t=Process_State."Error", s=w269, f=w271) -> (s? t:f=w293:T5)
          }
          frame "Prime System" {
            n127 = call "Update Cart Status.vi"("Selection"=status_update."Main Status", "error in (no error)"=w339, "String"="SDS Clearing wells and lines" ("Reagent"), "FP"=w344) -> ("error out"=w336:errorcluster)  [unwired: 7 in]
            n128 = call "Run Script.vi"("Script Name"="Drain All Wells" ("name or relative path"), "Main References"=w344, "error in (no error)"=w336) -> ("error out"=w348:errorcluster)  [unwired: 8 in]
            n129 = call "Update Cart Status.vi"("Selection"=status_update."Main Status", "error in (no error)"=w348, "String"="SDS Priming input lines" ("Reagent"), "FP"=w344) -> ("error out"=w346:errorcluster)  [unwired: 7 in]
            n130 = call "Run Script.vi"("Script Name"="Prime Input Lines" ("name or relative path"), "Main References"=w344, "error in (no error)"=w346) -> ("error out"=w341:errorcluster)  [unwired: 8 in]
            n131 = for {
              tunnel: w350 -> [w375] mode=indexing
              tunnel: [w374] -> w349 mode=indexing
              n132 = Bundle By Name(cluster=w375, "Primed"=TRUE) -> (w374:T6)
            }
            n133 = flat-sequence {
              tunnel: w343 -> [w372]
              tunnel: [w365] -> w342
              tunnel: w341 -> [w364]
              tunnel: [w363] -> w340
              frame #0 {
                n134 = Tick Count (ms)() -> (millisecond timer value=w363:u32)
                n135 = Subtract(x=w363, y=w372) -> (x-y=w360:u32)
                n136 = Divide(x=w360, y=u32 1000) -> (x/y=w362:dbl)
                n137 = call "Time Left Calc.vi"("Enum"=Time_elapsed."Update", "error in (no error)"=w364, "Time"=w362) -> ("error out"=w371:errorcluster)  [unwired: 6 in, 2 out]
                n138 = call "Time Left Calc.vi"("Enum"=Time_elapsed."Read", "error in (no error)"=w371) -> ("error out"=w369:errorcluster, "Time Left"=w370:u32)  [unwired: 7 in, 1 out]
                n139 = call "Time Left Calc.vi"("Enum"=Time_elapsed."Start", "error in (no error)"=w369, "Time"=w370) -> ("error out"=w365:errorcluster)  [unwired: 6 in, 2 out]
              }
            }
            n140 = Select(t=Process_State."Rinse Wells" ("State"), s=w356, f=Process_State."Idle" ("State")) -> (s? t:f=w359:T5)
          }
          frame "Rinse Wells" {
            n141 = call "Update Cart Status.vi"("Selection"=status_update."Main Status", "error in (no error)"=w396, "String"="SDS Draining Wells" ("Reagent"), "FP"=w380) -> ("error out"=w395:errorcluster)  [unwired: 7 in]
            n142 = call "Run Script.vi"("Script Name"="Drain All Wells" ("name or relative path"), "Main References"=w380, "error in (no error)"=w395) -> ("error out"=w381:errorcluster)  [unwired: 8 in]
            n143 = call "Update Cart Status.vi"("Selection"=status_update."Main Status", "error in (no error)"=w381, "String"="SDS Rinsing Syringe" ("Reagent"), "FP"=w380) -> ("error out"=w388:errorcluster)  [unwired: 7 in]
            n144 = for {
              N: 3 -> [_]
              tunnel: "Rinse Syringe" ("name or relative path") -> [w422]
              shift-right: [w421] -> w385
              shift-left: w388 -> [w423]
              tunnel: w380 -> [w420]
              n145 = call "Run Script.vi"("Script Name"=w422, "Main References"=w420, "error in (no error)"=w423) -> ("error out"=w421:errorcluster)  [unwired: 8 in]
            }
            n146 = call "Update Cart Status.vi"("Selection"=status_update."Main Status", "error in (no error)"=w385, "String"="SDS Rinsing all wells" ("Reagent"), "FP"=w380) -> ("error out"=w390:errorcluster)  [unwired: 7 in]
            n147 = for {
              N: 4 -> [_]
              shift-right: [w424] -> w377
              shift-left: w390 -> [w427]
              tunnel: w380 -> [w425]
              tunnel: "Rinse All Wells" ("Script Name") -> [w426]
              n148 = call "Run Script.vi"("Script Name"=w426, "Main References"=w425, "error in (no error)"=w427) -> ("error out"=w424:errorcluster)  [unwired: 8 in]
            }
            n149 = flat-sequence {
              tunnel: w379 -> [w419]
              tunnel: [w412] -> w378
              tunnel: w377 -> [w411]
              tunnel: [w410] -> w376
              frame #0 {
                n150 = Tick Count (ms)() -> (millisecond timer value=w410:u32)
                n151 = Subtract(x=w410, y=w419) -> (x-y=w407:u32)
                n152 = Divide(x=w407, y=u32 1000) -> (x/y=w409:dbl)
                n153 = call "Time Left Calc.vi"("Enum"=Time_elapsed."Update", "error in (no error)"=w411, "Time"=w409) -> ("error out"=w414:errorcluster)  [unwired: 6 in, 2 out]
                n154 = call "Time Left Calc.vi"("Enum"=Time_elapsed."Read", "error in (no error)"=w414) -> ("error out"=w417:errorcluster, "Time Left"=w416:u32)  [unwired: 7 in, 1 out]
                n155 = call "Time Left Calc.vi"("Enum"=Time_elapsed."Start", "error in (no error)"=w417, "Time"=w416) -> ("error out"=w412:errorcluster)  [unwired: 6 in, 2 out]
              }
            }
            n156 = Select(t=Process_State."PrePresTest" ("State"), s=w402, f=Process_State."Idle" ("State")) -> (s? t:f=w406:T5)
          }
          frame "Fill Wells" {
            # "Move to TW position if we are not doing liquid check"
            n157 = Index Array(array=w441, index=w445) -> (element=w444:T10)
            n158 = Unbundle By Name(w444) -> ("Reagent"=w435:string, "Bottle"=w443:T30)
            n159 = call "Update Cart Status.vi"("Selection"=status_update."Reagent", "error in (no error)"=w436, "String"=w435, "Array"=w434, "FP"=w432) -> ("error out"=w433:errorcluster)  [unwired: 6 in]
            n160 = case shown="\"Bottle 1\"" w443 {
              tunnel: [Bottles."Bottle 1" ("Bottle X") Bottles."Bottle 2" ("Bottle X") Bottles."Bottle 3" ("Bottle X") Bottles."H2O" ("Bottle X")] -> w438
              frame "Bottle 1" {
              }
              frame "Bottle 2" {
              }
              frame "Bottle 3" {
              }
              frame "Bottle 4" {
              }
            }
            n161 = for {
              N: 4 -> [_]
              tunnel: w434 -> [w480] mode=indexing
              tunnel: w438 -> [w481]
              shift-right: [w482] -> w442
              shift-left: w433 -> [w478]
              tunnel: w432 -> [w477]
              tunnel: w435 -> [w476]
              i -> [w479]
              n162 = case shown="True" w480 {
                tunnel: w478 -> [w483 w492]
                tunnel: w479 -> [_ w484]
                tunnel: [w483 w495] -> w482
                tunnel: w481 -> [_ w493]
                tunnel: w477 -> [_ w489]
                tunnel: w476 -> [_ w487]
                frame False {
                }
                frame True {
                  n163 = Increment(x=w484) -> (x+1=w486:i32)
                  n164 = Format Into String(format string="Filling well %d with %s", w486, w487) -> (resulting string=w485:string)  [unwired: 2 in, 1 out]
                  n165 = call "Update Cart Status.vi"("Selection"=status_update."Main Status", "error in (no error)"=w492, "String"=w485, "FP"=w489) -> ("error out"=w491:errorcluster)  [unwired: 7 in]
                  n166 = call "Run Script.vi"("Script Name"="Fill Well_X Reagent_X" ("name or relative path"), "Main References"=w489, "error in (no error)"=w491, "Drain X"=w484, "Well X"=w484, "Bottle X"=w493) -> ("error out"=w495:errorcluster)  [unwired: 5 in]
                }
              }
            }
            n167 = case shown="True" FALSE {
              tunnel: w442 -> [w467 w470]
              tunnel: [w467 w469] -> w429
              tunnel: w432 -> [_ w468]
              frame False {
              }
              frame True {
                n168 = call "Run Script.vi"("Script Name"="Move to TW" ("name or relative path"), "Main References"=w468, "error in (no error)"=w470) -> ("error out"=w469:errorcluster)  [unwired: 8 in]
              }
            }
            n169 = flat-sequence {
              tunnel: [w460] -> w431
              tunnel: [w459] -> w430
              tunnel: w429 -> [w455]
              tunnel: w428 -> [w454]
              frame #0 {
                n170 = Tick Count (ms)() -> (millisecond timer value=w459:u32)
                n171 = Subtract(x=w459, y=w454) -> (x-y=w456:u32)
                n172 = Divide(x=w456, y=u32 1000) -> (x/y=w458:dbl)
                n173 = call "Time Left Calc.vi"("Enum"=Time_elapsed."Update", "error in (no error)"=w455, "Time"=w458) -> ("error out"=w462:errorcluster)  [unwired: 6 in, 2 out]
                n174 = call "Time Left Calc.vi"("Enum"=Time_elapsed."Read", "error in (no error)"=w462) -> ("error out"=w465:errorcluster, "Time Left"=w464:u32)  [unwired: 7 in, 1 out]
                n175 = call "Time Left Calc.vi"("Enum"=Time_elapsed."Start", "error in (no error)"=w465, "Time"=w464) -> ("error out"=w460:errorcluster)  [unwired: 6 in, 2 out]
              }
            }
            n176 = Select(t=Process_State."Apply Pressure" ("State"), s=w449, f=Process_State."Idle" ("State")) -> (s? t:f=w447:T5)
            n177 = Select(t=Process_State."Error" ("State"), s=w429, f=w447) -> (s? t:f=w446:T5)
          }
          frame "PrePresTest" {
            n178 = Unbundle By Name(w513) -> ("Config"=w520:refnum<vi>)
            n179 = property class="Clust (strict)"(reference=w520) -> ("Value"=w519:T1)  [unwired: 1 in, 2 out]
            n180 = Unbundle By Name(w519) -> ("TW Position"=w514:dbl, "Load Position"=w507:dbl)
            n181 = call "Update Cart Status.vi"("Selection"=status_update."Main Status", "error in (no error)"=w522, "String"="Testing for leaks and clogs", "FP"=w513) -> ("error out"=w515:errorcluster)  [unwired: 7 in]
            n182 = call "Detect Transition to TW.vi"("Main References"=w513, "error in (no error)"=w515, "Cart Array"=w510) -> ("error out"=w505:errorcluster, "Analysis"=w508:T7[])  [unwired: 7 in]
            n183 = case shown="True" TRUE {
              tunnel: w508 -> [_ w555]
              tunnel: w508 -> [_ w554]
              tunnel: w510 -> [w550 w553]
              tunnel: w513 -> [_ w552]
              tunnel: [w550 w551] -> w499
              frame False {
              }
              frame True {
                n184 = for {
                  tunnel: w555 -> [w561] mode=indexing
                  tunnel: w554 -> [w559] mode=indexing
                  tunnel: w553 -> [w560] mode=indexing
                  tunnel: w552 -> [w558]
                  tunnel: [w556] -> w551 mode=indexing
                  i -> [w557]
                  n185 = case shown="True" w560 {
                    selector: w560 -> [w562 _]
                    tunnel: w561 -> [_ w578]
                    tunnel: w559 -> [_ w577]
                    tunnel: w558 -> [_ w574]
                    tunnel: w557 -> [_ w573]
                    tunnel: [w562 w571] -> w556
                    frame False {
                    }
                    frame True {
                      n186 = Unbundle By Name(w578) -> ("Pressure"=w576:bool)
                      n187 = Unbundle By Name(w577) -> ("Decay"=w564:bool, "Pressure"=w575:bool)
                      n188 = Increment(x=w573) -> (x+1=w570:i32)
                      n189 = And(x=w576, y=w575) -> (x .and. y?=w565:bool)
                      n190 = Select(t="Test Passed" ("String"), s=w564, f="Clog Detected" ("String")) -> (s? t:f=w567:string)
                      n191 = And(x=w565, y=w564) -> (x .and. y?=w563:bool)
                      n192 = Select(t=w567, s=w565, f="Pressure Level Fail" ("String")) -> (s? t:f=w572:string)
                      n193 = case shown="False" w563 {
                        selector: w563 -> [w580 w584]
                        tunnel: w574 -> [w583 _]
                        tunnel: w570 -> [w582 _]
                        tunnel: w572 -> [w581 _]
                        tunnel: [w580 w584] -> w571
                        frame False {
                          n194 = call "Update 1 Cart Status.vi"("Selection"=Update_Single_Cart."Cart Status", "FP"=w583, "String"=w581, "Cartridge"=w582) -> ()  [unwired: 7 in, 1 out]
                        }
                        frame True {
                        }
                      }
                    }
                  }
                }
              }
            }
            n195 = flat-sequence {
              tunnel: [w535] -> w504
              tunnel: [w534] -> w503
              tunnel: w505 -> [w530]
              tunnel: w502 -> [w529]
              frame #0 {
                n196 = Tick Count (ms)() -> (millisecond timer value=w534:u32)
                n197 = Subtract(x=w534, y=w529) -> (x-y=w531:u32)
                n198 = Divide(x=w531, y=u32 1000) -> (x/y=w533:dbl)
                n199 = call "Time Left Calc.vi"("Enum"=Time_elapsed."Update", "error in (no error)"=w530, "Time"=w533) -> ("error out"=w537:errorcluster)  [unwired: 6 in, 2 out]
                n200 = call "Time Left Calc.vi"("Enum"=Time_elapsed."Read", "error in (no error)"=w537) -> ("error out"=w540:errorcluster, "Time Left"=w539:u32)  [unwired: 7 in, 1 out]
                n201 = call "Time Left Calc.vi"("Enum"=Time_elapsed."Start", "error in (no error)"=w540, "Time"=w539) -> ("error out"=w535:errorcluster)  [unwired: 6 in, 2 out]
              }
            }
            n202 = case shown="True" w511 {
              tunnel: w514 -> [w544 _]
              tunnel: w504 -> [w543 w548]
              tunnel: [w542 w547] -> w506
              tunnel: w507 -> [_ w546]
              frame True {
                n203 = call "Zaber Manager.vi"("Action"=Mot_Stage_Mngr."Abs Move", "Value"=w544, "error in (no error)"=w543) -> ("error out"=w542:errorcluster)  [unwired: 6 in, 6 out]
              }
              frame False {
                n204 = call "Zaber Manager.vi"("Action"=Mot_Stage_Mngr."Abs Move", "Value"=w546, "error in (no error)"=w548) -> ("error out"=w547:errorcluster)  [unwired: 6 in, 6 out]
              }
            }
            n205 = for {
              N: 4 -> [_]
              tunnel: w517 -> [w589] mode=indexing
              tunnel: [w590] -> w516 mode=indexing
              tunnel: w518 -> [w585]
              tunnel: w508 -> [w586] mode=indexing
              n206 = Unbundle By Name(w589) -> ("Test Array Pre"=w588:T7[])
              n207 = Insert Into Array(array=w588, index=w585, new element=w586) -> (w587:T7[])
              n208 = Bundle By Name(cluster=w589, "Test Array Pre"=w587) -> (w590:T6)
            }
            n209 = Select(t=Process_State."Fill Wells" ("State"), s=w511, f=Process_State."Idle" ("State")) -> (s? t:f=w498:T5)
            n210 = Or Array Elements(Boolean array=w499) -> (logical OR=w500:bool)
            n211 = Select(t=w498, s=w500, f=Process_State."Abort" ("State")) -> (s? t:f=w496:T5)
            n212 = Select(t=Process_State."Error" ("State"), s=w506, f=w496) -> (s? t:f=w525:T5)
          }
          frame "Apply Pressure" {
            n213 = call "Update Cart Status.vi"("Selection"=status_update."Main Status", "error in (no error)"=w609, "String"="Applying pressure" ("Reagent"), "FP"=w597) -> ("error out"=w593:errorcluster)  [unwired: 7 in]
            n214 = Unbundle By Name(w597) -> ("Config"=w596:refnum<vi>)
            n215 = property class="Clust (strict)"(reference=w596) -> ("Value"=w595:T1)  [unwired: 1 in, 2 out]
            n216 = Unbundle By Name(w595) -> ("TW Position"=w591:dbl)
            n217 = Index Array(array=w615, index=w621) -> (element=w622:T10)
            n218 = call "Zaber Manager.vi"("Action"=Mot_Stage_Mngr."Abs Move", "Value"=w591, "error in (no error)"=w593) -> ("error out"=w592:errorcluster)  [unwired: 6 in, 6 out]
            n219 = Unbundle By Name(w622) -> ("Wash Time(s)"=w616:dbl)
            n220 = call "16CH Denkovi Manager.vi"("Action"=16CH_Denkovi_Mngr."Pres ON", "error in (no error)"=w592, "Relays In"=w605) -> ("error out"=w620:errorcluster)  [unwired: 6 in, 2 out]
            n221 = flat-sequence {
              tunnel: w620 -> [w632]
              tunnel: [w632] -> w619
              tunnel: [w631] -> w618
              frame #0 {
                n222 = Tick Count (ms)() -> (millisecond timer value=w631:u32)
              }
            }
            n223 = while {
              tunnel: w619 -> [w649]
              tunnel: [w643] -> w614
              tunnel: w618 -> [w654]
              tunnel: w617 -> [_]
              tunnel: w616 -> [w653]
              tunnel: w597 -> [w642]
              tunnel: w605 -> [w641]
              tunnel: [w634] -> w598
              stop <- w650 stop-if-true
              n224 = call "DAQ Manager.vi"("DAQ Mngr Action"=DAQ_Mngr."Analyze Pres&Vac", "error in (no error)"=w649) -> ("error out"=w648:errorcluster)  [unwired: 6 in, 7 out]
              n225 = flat-sequence {
                tunnel: w648 -> [w656]
                tunnel: [w656] -> w644
                tunnel: [w655] -> w634
                frame #0 {
                  n226 = Tick Count (ms)() -> (millisecond timer value=w655:u32)
                }
              }
              n227 = expression code="x*1000"(w653) -> (w640:dbl)
              n228 = Subtract(x=w634, y=w654) -> (x-y=w636:u32)
              n229 = Subtract(x=w640, y=w636) -> (x-y=w639:dbl)
              n230 = expression code="x/1000"(w636) -> (w635:u32)
              n231 = expression code="x/1000"(w639) -> (w638:dbl)
              n232 = global read "Main Globals.vi" "Cancel"() -> (w652:bool)
              n233 = call "Time Left Calc.vi"("Enum"=Time_elapsed."Update", "Time"=w635) -> ()  [unwired: 7 in, 3 out]
              n234 = Format Into String(format string="%.1f seconds", w638) -> (resulting string=w645:string)  [unwired: 2 in, 1 out]
              n235 = Greater?(x=w636, y=w640) -> (0:w651:bool)
              n236 = Compound Arithmetic op=OR(w651, w652) -> (w650:bool)
              n237 = call "Update Cart Status.vi"("Selection"=status_update."Cartridge", "error in (no error)"=w644, "String"=w645, "Array"=w641, "FP"=w642) -> ("error out"=w643:errorcluster)  [unwired: 6 in]
            }
            n238 = call "16CH Denkovi Manager.vi"("Action"=16CH_Denkovi_Mngr."Pres Vent&Close", "error in (no error)"=w614, "Relays In"=w605) -> ("error out"=w607:errorcluster)  [unwired: 6 in, 2 out]
            n239 = call "Update Cart Status.vi"("Selection"=status_update."Cartridge", "error in (no error)"=w607, "String"="TW in progress", "Array"=w605, "FP"=w597) -> ("error out"=w604:errorcluster)  [unwired: 6 in]
            n240 = call "Time Left Calc.vi"("Enum"=Time_elapsed."Read", "error in (no error)"=w604) -> ("error out"=w602:errorcluster, "Time Left"=w600:u32)  [unwired: 7 in, 1 out]
            n241 = call "Time Left Calc.vi"("Enum"=Time_elapsed."Start", "error in (no error)"=w602, "Time"=w600) -> ("error out"=w599:errorcluster)  [unwired: 6 in, 2 out]
            n242 = Select(t=Process_State."Drain&Rinse" ("State"), s=w627, f=Process_State."Idle" ("State")) -> (s? t:f=w625:T5)
            n243 = Select(t=Process_State."Error" ("State"), s=w599, f=w625) -> (s? t:f=w624:T5)
          }
          frame "PostPresTest" {
            n244 = Unbundle By Name(w671) -> ("Config"=w677:refnum<vi>)
            n245 = property class="Clust (strict)"(reference=w677) -> ("Value"=w676:T1)  [unwired: 1 in, 2 out]
            n246 = Unbundle By Name(w676) -> ("Load Position"=w672:dbl)
            n247 = call "Update Cart Status.vi"("Selection"=status_update."Main Status", "error in (no error)"=w679, "String"="Testing for leaks and clogs", "FP"=w671) -> ("error out"=w665:errorcluster)  [unwired: 7 in]
            n248 = call "Detect Transition to Load.vi"("Main References"=w671, "error in (no error)"=w665, "Cart Array"=w657) -> ("error out"=w663:errorcluster, "Analysis"=w664:T7[])  [unwired: 7 in]
            n249 = case shown="True" FALSE {
              tunnel: w664 -> [_ w711]
              tunnel: w664 -> [_ w710]
              tunnel: w657 -> [w706 w709]
              tunnel: w671 -> [_ w708]
              tunnel: [w706 w707] -> w670
              frame False {
              }
              frame True {
                n250 = for {
                  tunnel: w711 -> [w717] mode=indexing
                  tunnel: w710 -> [w715] mode=indexing
                  tunnel: w709 -> [w716] mode=indexing
                  tunnel: w708 -> [w714]
                  tunnel: [w712] -> w707 mode=indexing
                  i -> [w713]
                  n251 = case shown="True" w716 {
                    selector: w716 -> [w718 _]
                    tunnel: w717 -> [_ w736]
                    tunnel: w715 -> [_ w735]
                    tunnel: w714 -> [_ w730]
                    tunnel: w713 -> [_ w728]
                    tunnel: [w718 w724] -> w712
                    frame False {
                    }
                    frame True {
                      n252 = Unbundle By Name(w736) -> ("Transition"=w734:bool, "Pressure"=w732:bool)
                      n253 = Unbundle By Name(w735) -> ("Transition"=w733:bool, "Pressure"=w731:bool)
                      n254 = Increment(x=w728) -> (x+1=w723:i32)
                      n255 = And(x=w732, y=w731) -> (x .and. y?=w727:bool)
                      n256 = And(x=w734, y=w733) -> (x .and. y?=w726:bool)
                      n257 = Select(t="Test Passed" ("String"), s=w726, f="Clog Detected" ("String")) -> (s? t:f=w720:string)
                      n258 = And(x=w726, y=w727) -> (x .and. y?=w729:bool)
                      n259 = Select(t=w720, s=w727, f="Pressure Level Fail" ("String")) -> (s? t:f=w725:string)
                      n260 = case shown="False" w729 {
                        selector: w729 -> [w738 w742]
                        tunnel: w730 -> [w741 _]
                        tunnel: w723 -> [w740 _]
                        tunnel: w725 -> [w739 _]
                        tunnel: [w738 w742] -> w724
                        frame False {
                          n261 = call "Update 1 Cart Status.vi"("Selection"=Update_Single_Cart."Cart Status", "FP"=w741, "String"=w739, "Cartridge"=w740) -> ()  [unwired: 7 in, 1 out]
                        }
                        frame True {
                        }
                      }
                    }
                  }
                }
              }
            }
            n262 = call "16CH Denkovi Manager.vi"("Action"=16CH_Denkovi_Mngr."Pres Vent&Close", "error in (no error)"=w663, "Relays In"=w657) -> ("error out"=w661:errorcluster)  [unwired: 6 in, 2 out]
            n263 = flat-sequence {
              tunnel: [w694] -> w660
              tunnel: [w693] -> w659
              tunnel: w661 -> [w689]
              tunnel: w658 -> [w688]
              frame #0 {
                n264 = Tick Count (ms)() -> (millisecond timer value=w693:u32)
                n265 = Subtract(x=w693, y=w688) -> (x-y=w690:u32)
                n266 = Divide(x=w690, y=u32 1000) -> (x/y=w692:dbl)
                n267 = call "Time Left Calc.vi"("Enum"=Time_elapsed."Update", "error in (no error)"=w689, "Time"=w692) -> ("error out"=w696:errorcluster)  [unwired: 6 in, 2 out]
                n268 = call "Time Left Calc.vi"("Enum"=Time_elapsed."Read", "error in (no error)"=w696) -> ("error out"=w699:errorcluster, "Time Left"=w698:u32)  [unwired: 7 in, 1 out]
                n269 = call "Time Left Calc.vi"("Enum"=Time_elapsed."Start", "error in (no error)"=w699, "Time"=w698) -> ("error out"=w694:errorcluster)  [unwired: 6 in, 2 out]
              }
            }
            n270 = for {
              N: 4 -> [_]
              tunnel: w674 -> [w747] mode=indexing
              tunnel: [w748] -> w673 mode=indexing
              tunnel: w675 -> [w743]
              tunnel: w664 -> [w744] mode=indexing
              n271 = Unbundle By Name(w747) -> ("Test Array Post"=w746:T7[])
              n272 = Insert Into Array(array=w746, index=w743, new element=w744) -> (w745:T7[])
              n273 = Bundle By Name(cluster=w747, "Test Array Post"=w745) -> (w748:T6)
            }
            n274 = case shown="True" w666 {
              tunnel: w672 -> [_ w704]
              tunnel: w660 -> [w701 w703]
              tunnel: [w701 w702] -> w668
              frame False {
              }
              frame True {
                n275 = call "Zaber Manager.vi"("Action"=Mot_Stage_Mngr."Abs Move", "Value"=w704, "error in (no error)"=w703) -> ("error out"=w702:errorcluster)  [unwired: 6 in, 6 out]
              }
            }
            n276 = Select(t=Process_State."Drain&Rinse" ("State"), s=w666, f=Process_State."Idle" ("State")) -> (s? t:f=w683:T5)
            n277 = Select(t=Process_State."Error" ("State"), s=w668, f=w683) -> (s? t:f=w682:T5)
          }
          frame "Drain&Rinse" {
            n278 = call "Update Cart Status.vi"("Selection"=status_update."Main Status", "error in (no error)"=w759, "String"="Draining Wells", "FP"=w760) -> ("error out"=w758:errorcluster)  [unwired: 7 in]
            n279 = Unbundle By Name(w760) -> ("Config"=w770:refnum<vi>)
            n280 = property class="Clust (strict)"(reference=w770) -> ("Value"=w769:T1)  [unwired: 1 in, 2 out]
            n281 = Unbundle By Name(w769) -> ("Load Position"=w768:dbl)
            n282 = Index Array(array=w777, index=w779) -> (element=w785:T10)
            n283 = call "Zaber Manager.vi"("Action"=Mot_Stage_Mngr."Abs Move", "Value"=w768, "error in (no error)"=w758) -> ("error out"=w764:errorcluster)  [unwired: 6 in, 6 out]
            n284 = Unbundle By Name(w785) -> ("# of Rinses"=w754:i16)
            n285 = for {
              N: 4 -> [_]
              shift-right: [w806] -> w763
              shift-left: w764 -> [w807]
              tunnel: w765 -> [w805] mode=indexing
              tunnel: w760 -> [w803]
              tunnel: "Drain Well X" ("Script Name") -> [w802]
              i -> [w804]
              n286 = case shown="True" w805 {
                tunnel: w807 -> [w808 w813]
                tunnel: [w808 w811] -> w806
                tunnel: w804 -> [_ w812]
                tunnel: w803 -> [_ w810]
                tunnel: w802 -> [_ w809]
                frame False {
                }
                frame True {
                  n287 = call "Run Script.vi"("Script Name"=w809, "Main References"=w810, "error in (no error)"=w813, "Drain X"=w812, "Well X"=w812) -> ("error out"=w811:errorcluster)  [unwired: 6 in]
                }
              }
            }
            n288 = case shown="False" w755 {
              tunnel: w754 -> [_ w801]
              tunnel: [i16 1 ("# of Rinses") w801] -> w753
              frame False {
              }
              frame True {
              }
            }
            n289 = case shown="Default" w753 {
              selector: w753 -> [_ w818]
              tunnel: w765 -> [_ w821]
              tunnel: w763 -> [w814 w815]
              tunnel: w760 -> [_ w820]
              tunnel: [w814 w819] -> w752
              tunnel: "Rinse Well X step1" ("Script Name") -> [_ w817]
              tunnel: "Rinse Well X step3" ("Script Name") -> [_ w816]
              frame 0 {
                # "skip rinsing if # of rinses is 0"
              }
              frame Default {
                n290 = for {
                  N: w818 -> [w830]
                  tunnel: w821 -> [w822]
                  tunnel: w820 -> [w823]
                  shift-right: [w832] -> w819
                  shift-left: w815 -> [w835]
                  tunnel: w817 -> [w826]
                  tunnel: w816 -> [w825]
                  i -> [w828]
                  n291 = Increment(x=w828) -> (x+1=w827:i32)
                  n292 = Format Into String(format string="Rinsing wells %d/%d", w827, w830) -> (resulting string=w829:string)  [unwired: 2 in, 1 out]
                  n293 = call "Update Cart Status.vi"("Selection"=status_update."Main Status", "error in (no error)"=w835, "String"=w829, "FP"=w823) -> ("error out"=w834:errorcluster)  [unwired: 7 in]
                  n294 = for {
                    N: 4 -> [_]
                    shift-right: [w854] -> w824
                    shift-left: w834 -> [w855]
                    tunnel: w822 -> [w853] mode=indexing
                    tunnel: w823 -> [w851]
                    tunnel: w826 -> [w850]
                    i -> [w852]
                    n295 = case shown="True" w853 {
                      tunnel: w855 -> [w856 w861]
                      tunnel: [w856 w859] -> w854
                      tunnel: w852 -> [_ w860]
                      tunnel: w851 -> [_ w858]
                      tunnel: w850 -> [_ w857]
                      frame False {
                      }
                      frame True {
                        n296 = call "Run Script.vi"("Script Name"=w857, "Main References"=w858, "error in (no error)"=w861, "Drain X"=w860, "Well X"=w860) -> ("error out"=w859:errorcluster)  [unwired: 6 in]
                      }
                    }
                  }
                  n297 = for {
                    N: 4 -> [_]
                    shift-right: [w842] -> w832
                    shift-left: w824 -> [w843]
                    tunnel: w822 -> [w841] mode=indexing
                    tunnel: w823 -> [w839]
                    tunnel: w825 -> [w838]
                    i -> [w840]
                    n298 = case shown="True" w841 {
                      tunnel: w843 -> [w844 w849]
                      tunnel: [w844 w847] -> w842
                      tunnel: w840 -> [_ w848]
                      tunnel: w839 -> [_ w846]
                      tunnel: w838 -> [_ w845]
                      frame False {
                      }
                      frame True {
                        n299 = call "Run Script.vi"("Script Name"=w845, "Main References"=w846, "error in (no error)"=w849, "Drain X"=w848, "Well X"=w848) -> ("error out"=w847:errorcluster)  [unwired: 6 in]
                      }
                    }
                  }
                }
              }
            }
            n300 = Increment(x=w779) -> (x+1=w778:i32)
            n301 = Array Size(array=w777) -> (size(s)=w780:i32)
            n302 = Greater?(x=w780, y=w778) -> (0:w776:bool)
            n303 = flat-sequence {
              tunnel: [w793] -> w751
              tunnel: [w792] -> w750
              tunnel: w752 -> [w788]
              tunnel: w749 -> [w787]
              frame #0 {
                n304 = Tick Count (ms)() -> (millisecond timer value=w792:u32)
                n305 = Subtract(x=w792, y=w787) -> (x-y=w789:u32)
                n306 = Divide(x=w789, y=u32 1000) -> (x/y=w791:dbl)
                n307 = call "Time Left Calc.vi"("Enum"=Time_elapsed."Update", "error in (no error)"=w788, "Time"=w791) -> ("error out"=w795:errorcluster)  [unwired: 6 in, 2 out]
                n308 = call "Time Left Calc.vi"("Enum"=Time_elapsed."Read", "error in (no error)"=w795) -> ("error out"=w798:errorcluster, "Time Left"=w797:u32)  [unwired: 7 in, 1 out]
                n309 = call "Time Left Calc.vi"("Enum"=Time_elapsed."Start", "error in (no error)"=w798, "Time"=w797) -> ("error out"=w793:errorcluster)  [unwired: 6 in, 2 out]
              }
            }
            n310 = Select(t=Process_State."Fill Wells" ("State"), s=w776, f=Process_State."Dry" ("State")) -> (s? t:f=w774:T5)
            n311 = Select(t=w774, s=w755, f=Process_State."Idle") -> (s? t:f=w772:T5)
            n312 = Select(t=Process_State."Error" ("State"), s=w751, f=w772) -> (s? t:f=w781:T5)
          }
          frame "Dry" {
            n313 = Unbundle By Name(w868) -> ("Config"=w874:refnum<vi>)
            n314 = property class="Clust (strict)"(reference=w874) -> ("Value"=w872:T1)  [unwired: 1 in, 2 out]
            n315 = Unbundle By Name(w872) -> ("Dry Time(s)"=w871:dbl, "TW Position"=w873:dbl)
            n316 = Format Into String(format string="Drying capillaries for %ds", w871) -> (resulting string=w869:string)  [unwired: 2 in, 1 out]
            n317 = call "Update Cart Status.vi"("Selection"=status_update."Main Status", "error in (no error)"=w876, "String"=w869, "FP"=w868) -> ("error out"=w875:errorcluster)  [unwired: 7 in]
            n318 = call "Zaber Manager.vi"("Action"=Mot_Stage_Mngr."Abs Move", "Value"=w873, "error in (no error)"=w875) -> ("error out"=w882:errorcluster)  [unwired: 6 in, 6 out]
            n319 = call "16CH Denkovi Manager.vi"("Action"=16CH_Denkovi_Mngr."Pres ON", "error in (no error)"=w882, "Relays In"=w867) -> ("error out"=w894:errorcluster)  [unwired: 6 in, 2 out]
            n320 = flat-sequence {
              tunnel: w894 -> [w898]
              tunnel: [w898] -> w893
              tunnel: [w897] -> w892
              frame #0 {
                n321 = Tick Count (ms)() -> (millisecond timer value=w897:u32)
              }
            }
            n322 = while {
              tunnel: w893 -> [w915]
              tunnel: [w912] -> w890
              tunnel: w892 -> [w920]
              tunnel: w867 -> [w909]
              tunnel: w891 -> [_]
              tunnel: w871 -> [w919]
              tunnel: w868 -> [w910]
              tunnel: [w900] -> w862
              stop <- w916 stop-if-true
              n323 = call "DAQ Manager.vi"("DAQ Mngr Action"=DAQ_Mngr."Analyze Pres&Vac", "error in (no error)"=w915) -> ("error out"=w914:errorcluster)  [unwired: 6 in, 7 out]
              n324 = flat-sequence {
                tunnel: w914 -> [w922]
                tunnel: [w922] -> w913
                tunnel: [w921] -> w900
                frame #0 {
                  n325 = Tick Count (ms)() -> (millisecond timer value=w921:u32)
                }
              }
              n326 = expression code="x*1000"(w919) -> (w904:dbl)
              n327 = Subtract(x=w900, y=w920) -> (x-y=w903:u32)
              n328 = Subtract(x=w904, y=w903) -> (x-y=w908:dbl)
              n329 = expression code="x/1000"(w903) -> (w902:u32)
              n330 = expression code="x/1000"(w908) -> (w907:dbl)
              n331 = Greater?(x=w903, y=w904) -> (0:w917:bool)
              n332 = call "Time Left Calc.vi"("Enum"=Time_elapsed."Update", "Time"=w902) -> ()  [unwired: 7 in, 3 out]
              n333 = Format Into String(format string="%.1f seconds", w907) -> (resulting string=w905:string)  [unwired: 2 in, 1 out]
              n334 = global read "Main Globals.vi" "Cancel"() -> (w918:bool)
              n335 = call "Update Cart Status.vi"("Selection"=status_update."Cartridge", "error in (no error)"=w913, "String"=w905, "Array"=w909, "FP"=w910) -> ("error out"=w912:errorcluster)  [unwired: 6 in]
              n336 = Compound Arithmetic op=OR(w917, w918) -> (w916:bool)
            }
            n337 = call "16CH Denkovi Manager.vi"("Action"=16CH_Denkovi_Mngr."Pres Vent&Close", "error in (no error)"=w890, "Relays In"=w867) -> ("error out"=w863:errorcluster)  [unwired: 6 in, 2 out]
            n338 = Select(t=Process_State."Report" ("State"), s=w879, f=Process_State."Idle" ("State")) -> (s? t:f=w885:T5)
            n339 = call "Time Left Calc.vi"("Enum"=Time_elapsed."Start", "error in (no error)"=w863, "Time"=u32 0) -> ("error out"=w864:errorcluster)  [unwired: 6 in, 2 out]
            n340 = Select(t=Process_State."Error" ("State"), s=w864, f=w885) -> (s? t:f=w884:T5)
          }
          frame "Error" {
            # "TODO:  handle errors\nask user to remove cartridges"
            n341 = call "Data Logger.vi"("Action"=T16."Close", "error in"=w926) -> ("error out"=w925:errorcluster)  [unwired: 9 in]
            n342 = Unbundle By Name(w928) -> ("Cartridges"=w933:refnum<vi>)
            n343 = Unbundle By Name(w928) -> ("Start TW"=w935:refnum<vi>)
            n344 = property class="Bool (strict)"(reference=w935, "Value"=FALSE) -> ()  [unwired: 1 in, 2 out]
            n345 = property class="Clust (strict)"(reference=w933) -> (reference out=w930:refnum<vi>, "Value"=w932:T27)  [unwired: 1 in, 1 out]
            n346 = Bundle By Name(cluster=w932, "Current Status"="Error has occured.  Process aborted") -> (w929:T27)
            n347 = property class="Clust (strict)"(reference=w930, "Value"=w929) -> ()  [unwired: 1 in, 2 out]
          }
          frame "Abort" {
            n348 = call "Update Cart Status.vi"("Selection"=status_update."Main Status", "error in (no error)"=w962, "String"="Aborting Run" ("Reagent"), "FP"=w945) -> ("error out"=w952:errorcluster)  [unwired: 7 in]
            n349 = Unbundle By Name(w945) -> ("Start TW"=w944:refnum<vi>)
            n350 = property class="Bool (strict)"(reference=w944, "Value"=FALSE) -> ()  [unwired: 1 in, 2 out]
            n351 = call "Zaber Manager.vi"("Action"=Mot_Stage_Mngr."Home", "error in (no error)"=w952) -> ("error out"=w958:errorcluster)  [unwired: 7 in, 6 out]
            n352 = call "16CH Denkovi Manager.vi"("Action"=16CH_Denkovi_Mngr."Set Peristaltic", "error in (no error)"=w958, "Relays In"=bool[] [FALSE, FALSE, FALSE, FALSE, FALSE, FALSE, FALSE, FALSE, FALSE, FALSE, FALSE, FALSE, FALSE, FALSE, FALSE, FALSE]) -> ("error out"=w957:errorcluster)  [unwired: 6 in, 2 out]
            n353 = call "16CH Denkovi Manager.vi"("Action"=16CH_Denkovi_Mngr."Pres Vent&Close", "error in (no error)"=w957, "Relays In"=bool[] [TRUE, TRUE, TRUE, TRUE, FALSE, FALSE, FALSE, FALSE, FALSE, FALSE, FALSE, FALSE, FALSE, FALSE, FALSE, FALSE]) -> ("error out"=w956:errorcluster)  [unwired: 6 in, 2 out]
            n354 = call "Tecan Mngr.vi"("Mngr Action"=Tricon_Mngr."Start Pump", "Pump Data"=T23 {"Syringe Pos"=0, "Rate"=60.0, "Volume"=0.0, "Valve"=enum."Waste", "Action"=enum."Withdraw", "Move Type"=enum."Abs", "Init"=TRUE, "Empty Syr."=FALSE, "Full Fill"=FALSE, "Units"=enum."ul/s"}, "Pump Config"=w951, "error in (no error)"=w956) -> ("error out"=w948:errorcluster)  [unwired: 6 in, 5 out]
            n355 = call "DAQ Manager.vi"("DAQ Mngr Action"=DAQ_Mngr."Pinch Valve Disengage", "error in (no error)"=w948) -> ("error out"=w947:errorcluster)  [unwired: 6 in, 7 out]
            n356 = call "Data Logger.vi"("Action"=T16."Close", "error in"=w947) -> ("error out"=w954:errorcluster)  [unwired: 9 in]
          }
          frame "Report" {
            n357 = Get Date/Time String(date format (0)=enum16{"short", "long", "abbreviated"}."short") -> (date string=w986:string, time string=w985:string)  [unwired: 2 in]
            n358 = Concatenate Strings(w986, "   " ("string"), w985) -> (w983:string)
            n359 = for {
              tunnel: w982 -> [w1015] mode=indexing
              tunnel: w983 -> [w1014]
              tunnel: [w1013] -> w980 mode=indexing
              tunnel: w975 -> [w1012] mode=indexing
              n360 = case shown="True" w1012 {
                tunnel: w1015 -> [w1016 w1019]
                tunnel: w1014 -> [_ w1018]
                tunnel: [w1016 w1017] -> w1013
                frame False {
                }
                frame True {
                  n361 = Bundle By Name(cluster=w1019, "Finish Timestamp"=w1018) -> (w1017:T6)
                }
              }
            }
            n362 = call "Data Logger.vi"("Action"=T16."Close", "error in"=w979) -> ("error out"=w978:errorcluster)  [unwired: 9 in]
            n363 = for {
              N: 4 -> [_]
              tunnel: w978 -> [w998]
              tunnel: [w997] -> w981
              tunnel: w975 -> [w996] mode=indexing
              tunnel: w980 -> [w995] mode=indexing
              tunnel: w977 -> [w994]
              i -> [w993]
              n364 = case shown="True" w996 {
                tunnel: w998 -> [w999 w1011]
                tunnel: [w999 w1008] -> w997
                tunnel: w995 -> [_ w1010]
                tunnel: w994 -> [_ w1007]
                tunnel: w993 -> [_ w1005]
                frame False {
                }
                frame True {
                  n365 = call "Create Summary File.vi"("FP"=w1007, "error in"=w1011, "Report"=w1010) -> ("error out"=w1009:errorcluster, "Pres?"=w1000:bool)  [unwired: 5 in, 2 out]
                  n366 = Increment(x=w1005) -> (x+1=w1002:i32)
                  n367 = Select(t="Pass" ("String"), s=w1000, f="Clog" ("String")) -> (s? t:f=w1001:string)
                  n368 = call "Update 1 Cart Status.vi"("Selection"=Update_Single_Cart."Cart Reagent", "FP"=w1007, "error in (no error)"=w1009, "String"=w1001, "Cartridge"=w1002) -> ("error out"=w1008:errorcluster)  [unwired: 6 in]
                }
              }
            }
          }
          frame "Finish" {
            n369 = Unbundle By Name(w1024) -> ("Config"=w1030:refnum<vi>)
            n370 = Unbundle By Name(w1024) -> ("Start TW"=w1039:refnum<vi>)
            n371 = property class="Clust (strict)"(reference=w1030) -> ("Value"=w1029:T1)  [unwired: 1 in, 2 out]
            n372 = Unbundle By Name(w1029) -> ("Bottom Position"=w1028:dbl)
            n373 = Unbundle By Name(w1024) -> ("Main Clean Cart"=w1025:refnum<vi>)
            n374 = property class="Bool (strict)"(reference=w1039, "Value"=FALSE) -> ()  [unwired: 1 in, 2 out]
            n375 = property class="Bool (strict)"(reference=w1025, "Value"=FALSE, "DisabledEnum"=T13."Enabled" ("Disabled")) -> ()  [unwired: 1 in, 2 out]
            n376 = call "Zaber Manager.vi"("Action"=Mot_Stage_Mngr."Abs Move", "Value"=w1028, "error in (no error)"=w1041) -> ("error out"=w1022:errorcluster)  [unwired: 6 in, 6 out]
            n377 = call "DAQ Manager.vi"("DAQ Mngr Action"=DAQ_Mngr."Pinch Valve Disengage", "error in (no error)"=w1022) -> ("error out"=w1021:errorcluster)  [unwired: 6 in, 7 out]
            n378 = call "Update Cart Status.vi"("Selection"=status_update."Cartridge", "error in (no error)"=w1021, "String"="Finished", "Array"=w1042, "FP"=w1024) -> ("error out"=w1034:errorcluster)  [unwired: 6 in]
            n379 = call "Update Cart Status.vi"("Selection"=status_update."Main Status", "error in (no error)"=w1034, "String"="Thermal Wash is finished, please remove catridges" ("Current Status"), "FP"=w1024) -> ("error out"=w1033:errorcluster)  [unwired: 7 in]
          }
          frame "-rinse wells" {
            n380 = call "Update Cart Status.vi"("Selection"=status_update."Main Status", "error in (no error)"=w1059, "String"="Draining All Wells and Lines", "FP"=w1052) -> ("error out"=w1058:errorcluster)  [unwired: 7 in]
            n381 = Unbundle By Name(w1052) -> ("Config"=w1065:refnum<vi>)
            n382 = property class="Clust (strict)"(reference=w1065) -> ("Value"=w1064:T1)  [unwired: 1 in, 2 out]
            n383 = Unbundle By Name(w1064) -> ("Load Position"=w1063:dbl)
            n384 = call "Zaber Manager.vi"("Action"=Mot_Stage_Mngr."Abs Move", "Value"=w1063, "error in (no error)"=w1058) -> ("error out"=w1062:errorcluster)  [unwired: 6 in, 6 out]
            n385 = call "Run Script.vi"("Script Name"="Drain All Wells", "Main References"=w1052, "error in (no error)"=w1062) -> ("error out"=w1053:errorcluster)  [unwired: 8 in]
            n386 = for {
              N: w1054 -> [w1076]
              shift-right: [w1079] -> w1050
              shift-left: w1053 -> [w1075]
              tunnel: w1052 -> [w1073]
              tunnel: w1052 -> [w1072]
              i -> [w1078]
              n387 = Format Into String(format string="Rinse %d of %d", w1078, w1076) -> (resulting string=w1074:string)  [unwired: 2 in, 1 out]
              n388 = call "Update Cart Status.vi"("Selection"=status_update."Main Status", "error in (no error)"=w1075, "String"=w1074, "FP"=w1073) -> ("error out"=w1080:errorcluster)  [unwired: 7 in]
              n389 = call "Run Script.vi"("Script Name"="Rinse All Wells", "Main References"=w1072, "error in (no error)"=w1080) -> ("error out"=w1079:errorcluster)  [unwired: 8 in]
            }
            n390 = Select(t=Process_State."Error" ("State"), s=w1050, f=Process_State."Idle" ("State")) -> (s? t:f=w1069:T5)
          }
          frame "-fill well" {
            # "Move to TW position if we are not doing liquid check"
            n391 = Unbundle By Name(w1095) -> ("Commands"=w1094:refnum<vi>)
            n392 = property class="Clust (strict)"(reference=w1094) -> ("Value"=w1093:T31)  [unwired: 1 in, 2 out]
            n393 = Unbundle By Name(w1093) -> ("Well #"=w1085:T32, "Bottle #"=w1086:T19)
            n394 = Format Into String(format string="Filling %s with %s", w1085, w1086) -> (resulting string=w1087:string)  [unwired: 2 in, 1 out]
            n395 = call "Update Cart Status.vi"("Selection"=status_update."Main Status", "error in (no error)"=w1092, "String"=w1087, "FP"=w1095) -> ("error out"=w1090:errorcluster)  [unwired: 7 in]
            n396 = call "Run Script.vi"("Script Name"="Fill Well_X Reagent_X" ("name or relative path"), "Main References"=w1095, "error in (no error)"=w1090, "Well X"=w1085, "Bottle X"=w1086) -> ("error out"=w1084:errorcluster)  [unwired: 6 in]
            n397 = Select(t=Process_State."PrePresTest" ("State"), s=w1103, f=Process_State."Idle" ("State")) -> (s? t:f=w1101:T5)
            n398 = Select(t=Process_State."Error" ("State"), s=w1084, f=w1101) -> (s? t:f=w1100:T5)
          }
          frame "-drain all" {
            # "Move to TW position if we are not doing liquid check"
            n399 = Unbundle By Name(w1118) -> ("Commands"=w1117:refnum<vi>)
            n400 = property class="Clust (strict)"(reference=w1117) -> ("Value"=w1116:T31)  [unwired: 1 in, 2 out]
            n401 = Unbundle By Name(w1116) -> ("Well #"=w1110:T32, "Bottle #"=w1111:T19)
            n402 = call "Update Cart Status.vi"("Selection"=status_update."Main Status", "error in (no error)"=w1115, "String"="Draining all wells" ("format string"), "FP"=w1118) -> ("error out"=w1113:errorcluster)  [unwired: 7 in]
            n403 = call "Run Script.vi"("Script Name"="Drain All Wells" ("name or relative path"), "Main References"=w1118, "error in (no error)"=w1113, "Well X"=w1110, "Bottle X"=w1111) -> ("error out"=w1109:errorcluster)  [unwired: 6 in]
            n404 = Select(t=Process_State."PrePresTest" ("State"), s=w1126, f=Process_State."Idle" ("State")) -> (s? t:f=w1124:T5)
            n405 = Select(t=Process_State."Error" ("State"), s=w1109, f=w1124) -> (s? t:f=w1123:T5)
          }
          frame "-clean cartridge" {
            # "clean time"
            # "TODO:  do all of this with one script\nneed to add Pressure X to script handler"
            n406 = call "Update Cart Status.vi"("Selection"=status_update."Main Status", "error in (no error)"=w1176, "String"="Cleaning cartridge", "FP"=w1146) -> ("error out"=w1144:errorcluster)  [unwired: 7 in]
            n407 = call "DAQ Manager.vi"("DAQ Mngr Action"=DAQ_Mngr."Pinch Valve Engage", "error in (no error)"=w1144) -> ("error out"=w1143:errorcluster)  [unwired: 6 in, 7 out]
            n408 = for {
              shift-right: [w1198] -> w1159
              shift-left: w1143 -> [w1199]
              tunnel: w1146 -> [w1197]
              tunnel: w1130 -> [w1196] mode=indexing
              tunnel: "Drain Well X" ("name or relative path") -> [w1195]
              i -> [w1194]
              n409 = case shown="True" w1196 {
                tunnel: w1199 -> [w1200 w1205]
                tunnel: [w1200 w1203] -> w1198
                tunnel: w1197 -> [_ w1204]
                tunnel: w1195 -> [_ w1202]
                tunnel: w1194 -> [_ w1201]
                frame False {
                }
                frame True {
                  n410 = call "Run Script.vi"("Script Name"=w1202, "Main References"=w1204, "error in (no error)"=w1205, "Drain X"=w1201, "Well X"=w1201) -> ("error out"=w1203:errorcluster)  [unwired: 6 in]
                }
              }
            }
            n411 = Unbundle By Name(w1146) -> ("Commands"=w1174:refnum<vi>)
            n412 = Unbundle By Name(w1146) -> ("Config"=w1165:refnum<vi>)
            n413 = property class="Clust (strict)"(reference=w1165) -> ("Value"=w1164:T1)  [unwired: 1 in, 2 out]
            n414 = Unbundle By Name(w1164) -> ("Bottom Position"=w1137:dbl, "TW Position"=w1151:dbl, "Dry Time(s)"=w1149:dbl)
            n415 = property class="Clust (strict)"(reference=w1174) -> (reference out=w1168:refnum<vi>, "Value"=w1170:T31)  [unwired: 1 in, 1 out]
            n416 = for {
              shift-right: [w1185] -> w1157
              shift-left: w1159 -> [w1186]
              tunnel: w1146 -> [w1184]
              tunnel: w1130 -> [w1183] mode=indexing
              tunnel: "Fill Well_X Reagent_X" ("name or relative path") -> [w1182]
              i -> [w1181]
              n417 = case shown="True" w1183 {
                tunnel: w1186 -> [w1187 w1193]
                tunnel: [w1187 w1191] -> w1185
                tunnel: w1184 -> [_ w1192]
                tunnel: w1182 -> [_ w1190]
                tunnel: w1181 -> [_ w1189]
                frame False {
                }
                frame True {
                  n418 = call "Run Script.vi"("Script Name"=w1190, "Main References"=w1192, "error in (no error)"=w1193, "Drain X"=w1189, "Well X"=w1189, "Bottle X"=Bottles."H2O") -> ("error out"=w1191:errorcluster)  [unwired: 5 in]
                }
              }
            }
            n419 = call "Zaber Manager.vi"("Action"=Mot_Stage_Mngr."Abs Move", "Value"=w1151, "error in (no error)"=w1157) -> ("error out"=w1155:errorcluster)  [unwired: 6 in, 6 out]
            n420 = Bundle By Name(cluster=w1170, "Clean&Dry Cartridge"=FALSE ("Check for leaks")) -> (w1167:T31)
            n421 = call "16CH Denkovi Manager.vi"("Action"=16CH_Denkovi_Mngr."Pres ON", "error in (no error)"=w1155, "Relays In"=w1130) -> ("error out"=w1152:errorcluster)  [unwired: 6 in, 2 out]
            n422 = call "Delay with Cancel 2.vi"("Insert Error"=FALSE, "error in (no error)"=w1152, "Delay(s)"=180.0) -> ("error out"=w1140:errorcluster)  [unwired: 7 in, 1 out]
            n423 = for {
              shift-right: [w1210] -> w1133
              shift-left: w1140 -> [w1211]
              tunnel: w1146 -> [w1209]
              tunnel: w1130 -> [w1208] mode=indexing
              tunnel: "Drain Well X" ("name or relative path") -> [w1207]
              i -> [w1206]
              n424 = case shown="True" w1208 {
                tunnel: w1211 -> [w1212 w1217]
                tunnel: [w1212 w1215] -> w1210
                tunnel: w1209 -> [_ w1216]
                tunnel: w1207 -> [_ w1214]
                tunnel: w1206 -> [_ w1213]
                frame False {
                }
                frame True {
                  n425 = call "Run Script.vi"("Script Name"=w1214, "Main References"=w1216, "error in (no error)"=w1217, "Drain X"=w1213, "Well X"=w1213) -> ("error out"=w1215:errorcluster)  [unwired: 6 in]
                }
              }
            }
            n426 = call "16CH Denkovi Manager.vi"("Action"=16CH_Denkovi_Mngr."Pres ON", "error in (no error)"=w1133, "Relays In"=w1130) -> ("error out"=w1132:errorcluster)  [unwired: 6 in, 2 out]
            n427 = call "Delay with Cancel 2.vi"("Insert Error"=FALSE, "error in (no error)"=w1132, "Delay(s)"=w1149) -> ("error out"=w1136:errorcluster)  [unwired: 7 in, 1 out]
            n428 = call "DAQ Manager.vi"("DAQ Mngr Action"=DAQ_Mngr."Pinch Valve Disengage", "error in (no error)"=w1136) -> ("error out"=w1134:errorcluster)  [unwired: 6 in, 7 out]
            n429 = call "16CH Denkovi Manager.vi"("Action"=16CH_Denkovi_Mngr."Pres Vent&Close", "error in (no error)"=w1134, "Relays In"=w1130) -> ("error out"=w1135:errorcluster)  [unwired: 6 in, 2 out]
            n430 = call "Zaber Manager.vi"("Action"=Mot_Stage_Mngr."Abs Move", "Value"=w1137, "error in (no error)"=w1135) -> ("error out"=w1139:errorcluster)  [unwired: 6 in, 6 out]
            n431 = property class="Clust (strict)"(reference=w1168, error in=w1139, "Value"=w1167) -> (error out=w1163:errorcluster)  [unwired: 1 out]
            n432 = Select(t=Process_State."Error" ("State"), s=w1163, f=Process_State."Idle" ("State")) -> (s? t:f=w1179:T5)
          }
          frame "-check cartridge" {
            n433 = call "Update Cart Status.vi"("Selection"=status_update."Main Status", "error in (no error)"=w1249, "String"="Checking cartridge", "FP"=w1236) -> ("error out"=w1223:errorcluster)  [unwired: 7 in]
            n434 = call "DAQ Manager.vi"("DAQ Mngr Action"=DAQ_Mngr."Pinch Valve Engage", "error in (no error)"=w1223) -> ("error out"=w1222:errorcluster)  [unwired: 6 in, 7 out]
            n435 = Unbundle By Name(w1236) -> ("Commands"=w1247:refnum<vi>)
            n436 = disable-structure shown="Enabled" {
              disable-tunnel: [w1273 w1288] -> w1243
              disable-tunnel: w1236 -> [w1272 _]
              disable-tunnel: w1226 -> [w1271 _]
              disable-tunnel: w1222 -> [w1270 w1288]
              frame Disabled {
                n437 = for {
                  shift-right: [w1277] -> w1273
                  shift-left: w1270 -> [w1278]
                  tunnel: w1272 -> [w1276]
                  tunnel: w1271 -> [w1275] mode=indexing
                  i -> [w1274]
                  n438 = case shown="True" w1275 {
                    tunnel: w1278 -> [w1279 w1285]
                    tunnel: [w1279 w1283] -> w1277
                    tunnel: w1276 -> [_ w1282]
                    tunnel: w1274 -> [_ w1280]
                    frame False {
                    }
                    frame True {
                      n439 = call "Run Script.vi"("Script Name"="Drain Well X" ("name or relative path"), "Main References"=w1282, "error in (no error)"=w1285, "Drain X"=w1280, "Well X"=w1280) -> ("error out"=w1284:errorcluster)  [unwired: 6 in]
                      n440 = call "Run Script.vi"("Script Name"="Fill Well_X Reagent_X" ("name or relative path"), "Main References"=w1282, "error in (no error)"=w1284, "Drain X"=w1280, "Well X"=w1280, "Bottle X"=Bottles."H2O") -> ("error out"=w1283:errorcluster)  [unwired: 5 in]
                    }
                  }
                }
              }
              frame Enabled {
              }
            }
            n441 = Unbundle By Name(w1236) -> ("Config"=w1235:refnum<vi>)
            n442 = property class="Clust (strict)"(reference=w1235) -> ("Value"=w1234:T1)  [unwired: 1 in, 2 out]
            n443 = property class="Clust (strict)"(reference=w1247) -> (reference out=w1240:refnum<vi>, "Value"=w1242:T31)  [unwired: 1 in, 1 out]
            n444 = Unbundle By Name(w1234) -> ("Bottom Position"=w1233:dbl)
            n445 = call "Detect Transition to TW.vi"("Main References"=w1236, "error in (no error)"=w1243, "Cart Array"=w1226) -> ("error out"=w1228:errorcluster, "Analysis"=w1229:T7[])  [unwired: 7 in]
            n446 = call "16CH Denkovi Manager.vi"("Action"=16CH_Denkovi_Mngr."Pres Vent&Close", "error in (no error)"=w1228, "Relays In"=w1226) -> ("error out"=w1227:errorcluster)  [unwired: 6 in, 2 out]
            n447 = Bundle By Name(cluster=w1242, "Check for leaks"=FALSE, "Cart Test Array"=w1229) -> (w1239:T31)
            n448 = call "Zaber Manager.vi"("Action"=Mot_Stage_Mngr."Abs Move", "Value"=w1233, "error in (no error)"=w1227) -> ("error out"=w1220:errorcluster)  [unwired: 6 in, 6 out]
            n449 = call "DAQ Manager.vi"("DAQ Mngr Action"=DAQ_Mngr."Pinch Valve Disengage", "error in (no error)"=w1220) -> ("error out"=w1219:errorcluster)  [unwired: 6 in, 7 out]
            n450 = disable-structure shown="Enabled" {
              disable-tunnel: w1219 -> [w1257 w1269]
              disable-tunnel: w1236 -> [w1256 _]
              disable-tunnel: [w1255 w1269] -> w1232
              disable-tunnel: w1226 -> [w1254 _]
              frame Disabled {
                n451 = for {
                  shift-right: [w1261] -> w1255
                  shift-left: w1257 -> [w1262]
                  tunnel: w1256 -> [w1260]
                  tunnel: w1254 -> [w1259] mode=indexing
                  i -> [w1258]
                  n452 = case shown="True" w1259 {
                    tunnel: w1262 -> [w1263 w1267]
                    tunnel: [w1263 w1265] -> w1261
                    tunnel: w1260 -> [_ w1266]
                    tunnel: w1258 -> [_ w1264]
                    frame False {
                    }
                    frame True {
                      n453 = call "Run Script.vi"("Script Name"="Drain Well X" ("name or relative path"), "Main References"=w1266, "error in (no error)"=w1267, "Drain X"=w1264, "Well X"=w1264) -> ("error out"=w1265:errorcluster)  [unwired: 6 in]
                    }
                  }
                }
              }
              frame Enabled {
              }
            }
            n454 = property class="Clust (strict)"(reference=w1240, error in=w1232, "Value"=w1239) -> (error out=w1231:errorcluster)  [unwired: 1 out]
            n455 = Select(t=Process_State."Error" ("State"), s=w1231, f=Process_State."Idle" ("State")) -> (s? t:f=w1252:T5)
          }
        }
      }
    }
    frame Error {
      (unwired) T33 {"negative limit switch"=FALSE, "positive limit switch"=FALSE, "home switch"=FALSE, "position marker"=FALSE, "device enable"=FALSE, "quick stop"=FALSE, "general purpose J"=FALSE, "general purpose I"=FALSE, "general purpose H"=FALSE, "general purpose G"=FALSE, "general purpose F"=FALSE, "general purpose E"=FALSE, "general purpose D"=FALSE, "general purpose C"=FALSE, "general purpose B"=FALSE, "general purpose A"=FALSE} ("digital inputs")
    }
  }
  "error out" <- w11
  "Wash Array" <- w6
  "State Out" <- w7
  "Reports" <- w4
